vi "接口测试_20190220.vi"() -> ()   [LabVIEW 2017]
uses:
  D:/QuiKLab3.0/QuiKLabAPI.dll
panel:
  in  "启动任务":bool
  out "双击":string
  out "信号":string
  out "获取订阅的信号参数值":dbl
  in  "卸载工程 2":bool
  in  "用例运行状态":i32(listbox)
  in  "任务下用例状态":i32(listbox)
  in  "用例分类下用例":i32(listbox)
  in  "用例分类":i32(listbox)
  in  "任务分类下任务":i32(listbox)
  in  "测试任务":i32(listbox) caption="测试任务分类"
  in  "测试用例":i32(listbox)
  out "文件数量":i32
  in  "运行时参数列表":i32(listbox)
  in  "板卡设备IP":string
  out "板卡信息列表":i32(listbox)
  in  "设置的内容":string
  out "设置文件内容结果":i32
  in  "设置文件内容":bool
  out "显示的内容":string
  in  "目录":i32(listbox)=-1
  out "获取选中参数值":dbl
  in  "输入设备IP":string
  in  "下位机信息":bool
  out "下位机列表":i32(listbox)
  out "IP是否在线":i32
  out "更新信息是否成功":i32
  out "板卡类型个数":i32
  in  "字符串 3":string="00000000000000000000000000000000000000000000000000000000000000000000000000000000000000"
  out "下位机个数":i32
  in  "获得初始值列表":i32(listbox)
  in  "获得初始值":bool
  in  "输出信号列表":string(tree)
  in  "输出信号参数列表":bool
  out "项目个数":i32
  in  "工程选择：":i32(listbox)
  in  "字符串":string="00000000000000000000000000000000000000000000000000000000000000000000000000000000000000"
  in  "输入信号参数列表":bool
  in  "输入信号列表":string(tree)
  out "取消订阅":i32
  out "使用下位机返回值":i32
  in  "停止测试用例":bool
  out "StartTest":i32
  out "useTestCase":i32
  in  "执行用例":bool
  out "刷新返回结果":i32
  out "设置初始值结果":i32
  in  "设置初始值":bool
  out "发送信号结果":i32
  in  "发送信号":bool
  out "输出信号参数值":dbl
  in  "输出信号参数值":dbl
  in  "设置输出信号参数值":bool
  out "设置输出参数值":i32
  out "重置参数值":i32
  out "获取输入订阅信号参数值":dbl
  in  "重置按钮":bool
  in  "获取用例集列表":bool
  out "用例集":string(tree)
  in  "获取任务集列表":bool
  in  "任务集":string(tree)
  out "当前工程名称":string
  out "卸载工程结果":i32
  in  "卸载工程":bool
  in  "更新路径":bool
  in  "加载工程":bool
  out "导出用例相关信息结果":i32
  in  "导出工程用例相关信息":bool
  out "设置实时参数值返回值":i32
  in  "设置实时参数值":dbl
  in  "设置参数值":bool
  out "暂停和继续结果":i32
  in  "暂停按钮":bool
  out "停止任务集结果 2":i32
  out "波形图表":dbl(graph)
  in  "退出程序":bool
  in  "媒体停止按钮":bool
  in  "播放按钮":bool
  out "释放平台结果":i32
  out "卸载工程结果 2":i32
  out "停止测试用例":i32
  out "开始任务集":i32
  out "加载工程结果":i32
  out "初始化平台结果":i32
  out "错误输出":errorcluster
  out "更新路径结果":i32
  # "下位机信息"
  # "文件操作"
  # "平台初始化"
  # "测试任务执行"
  # "测试用例执行"
  # "实时监视"
  # "信号"
  # "初始值"
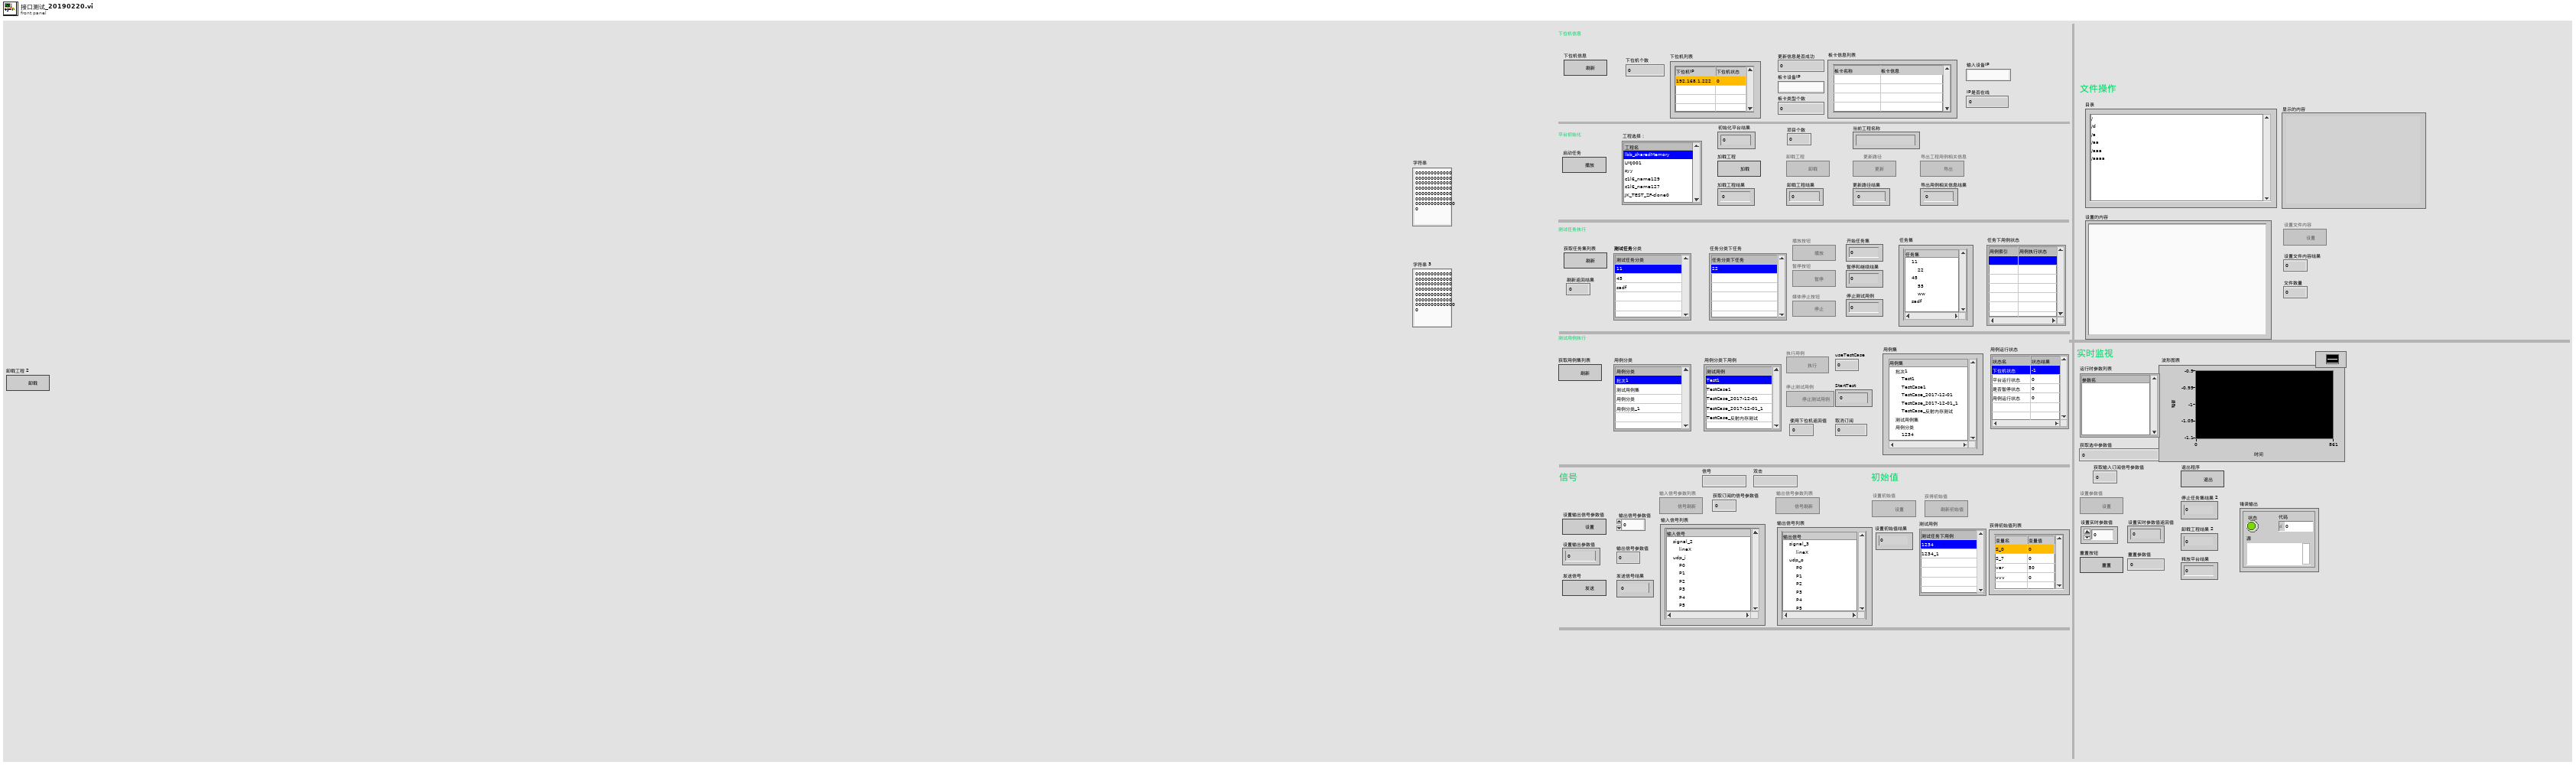
[diagram p1: front panel]
types:
  T1 = enum8{"loadPro", "unLoadPro", "updatePath", "export", "play", "pause", "stop"}
  T2 = enum8{"Enabled", "Disabled", "Disabled and Grayed Out"}
  T3 = enum8{"Enabled", "Disabled", "Disabled and Grayed Out", ""}
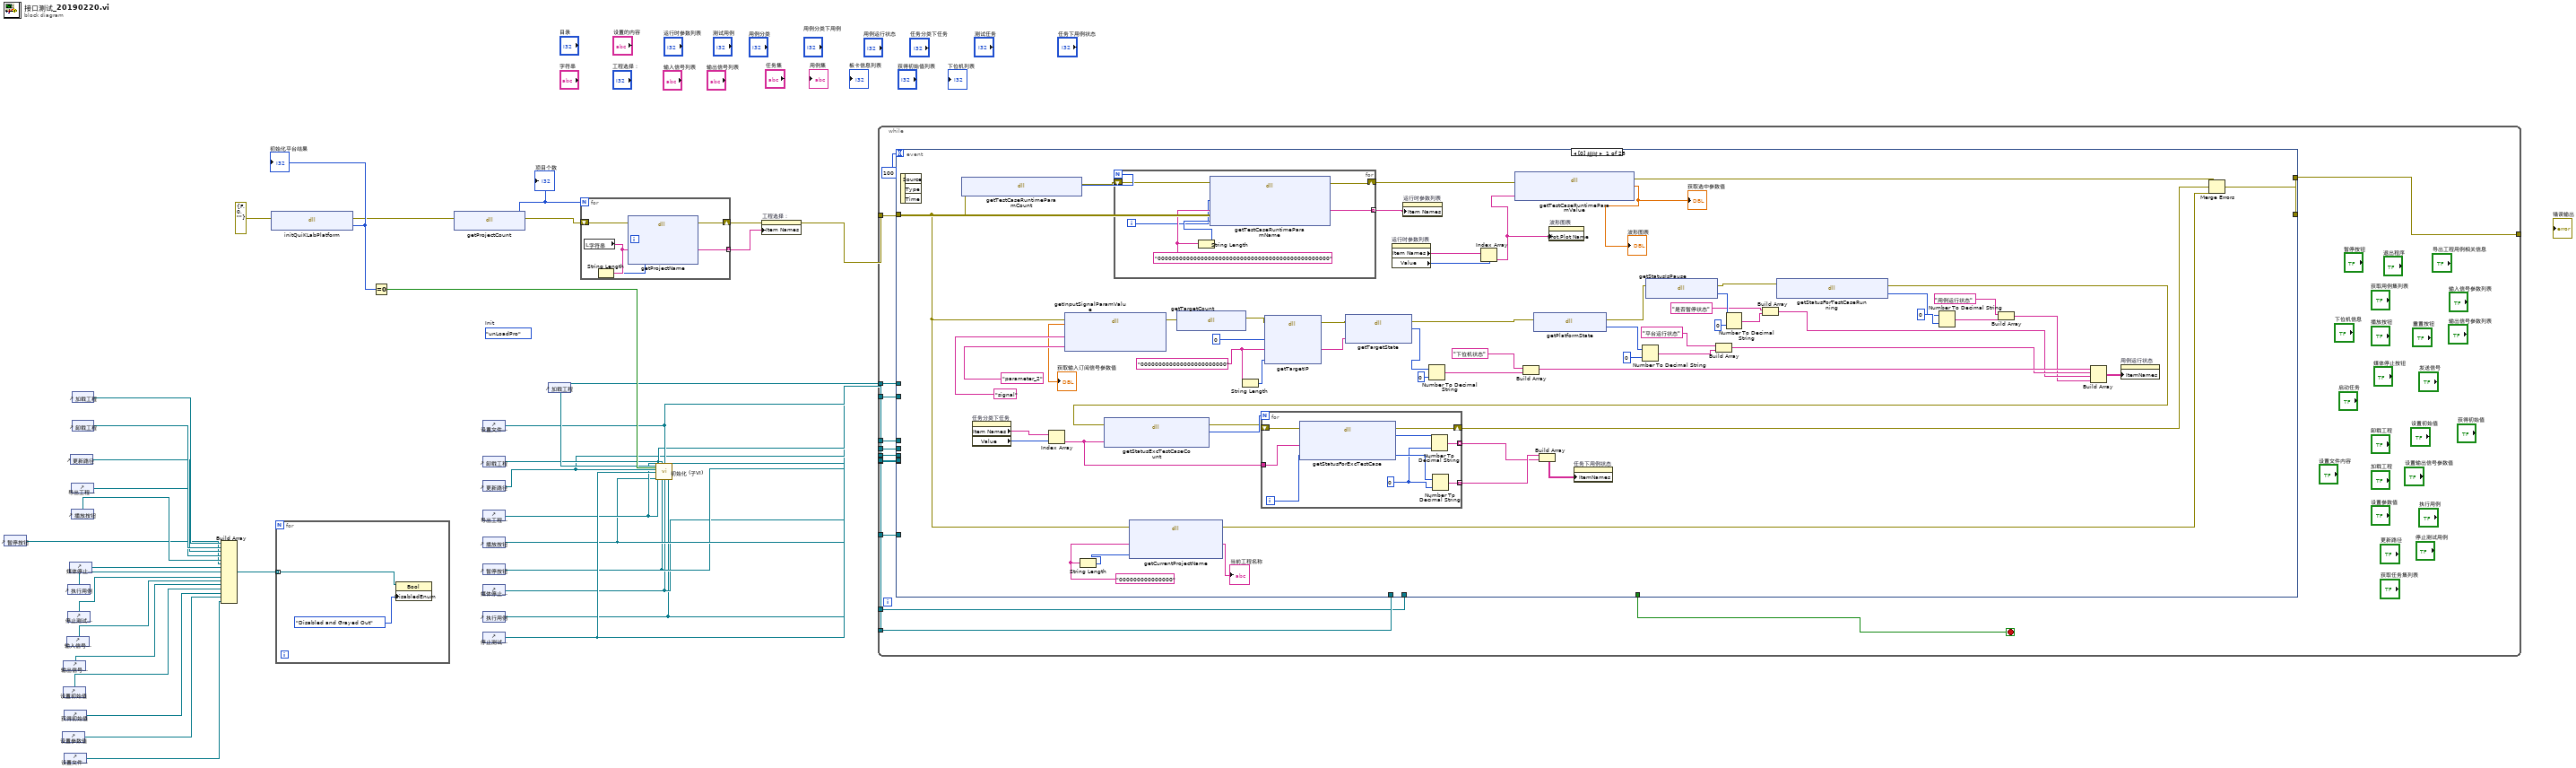
[diagram p0: block diagram]
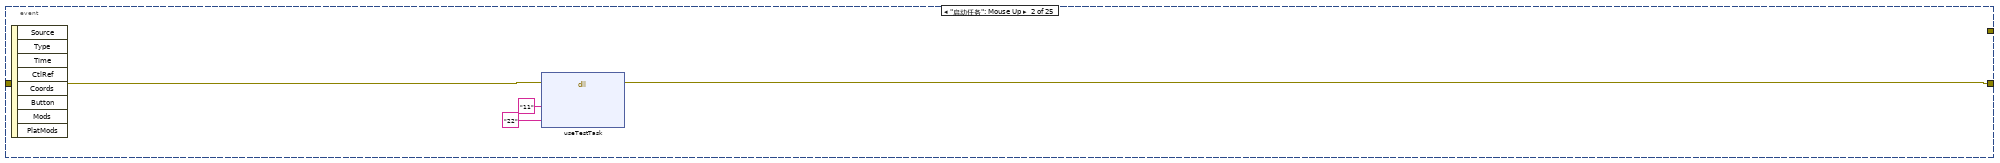
[diagram p2: hidden frame]
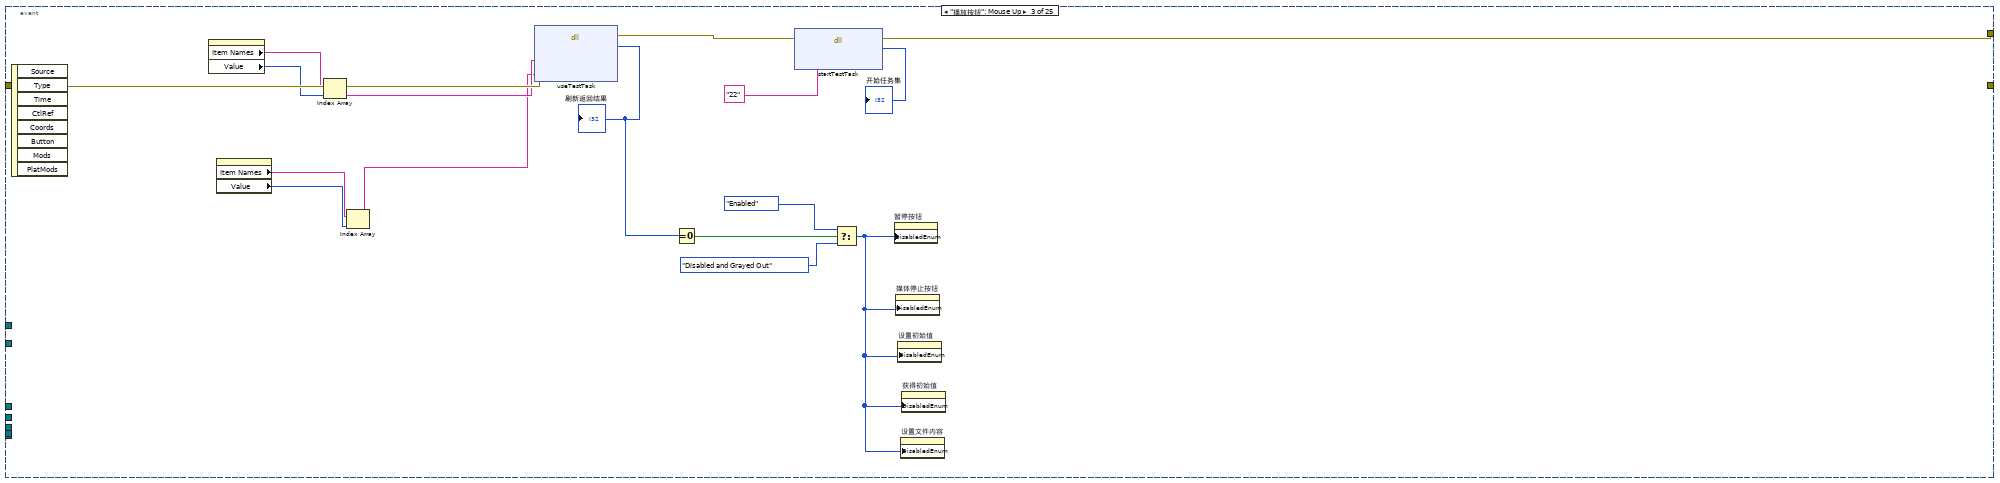
[diagram p3: hidden frame]
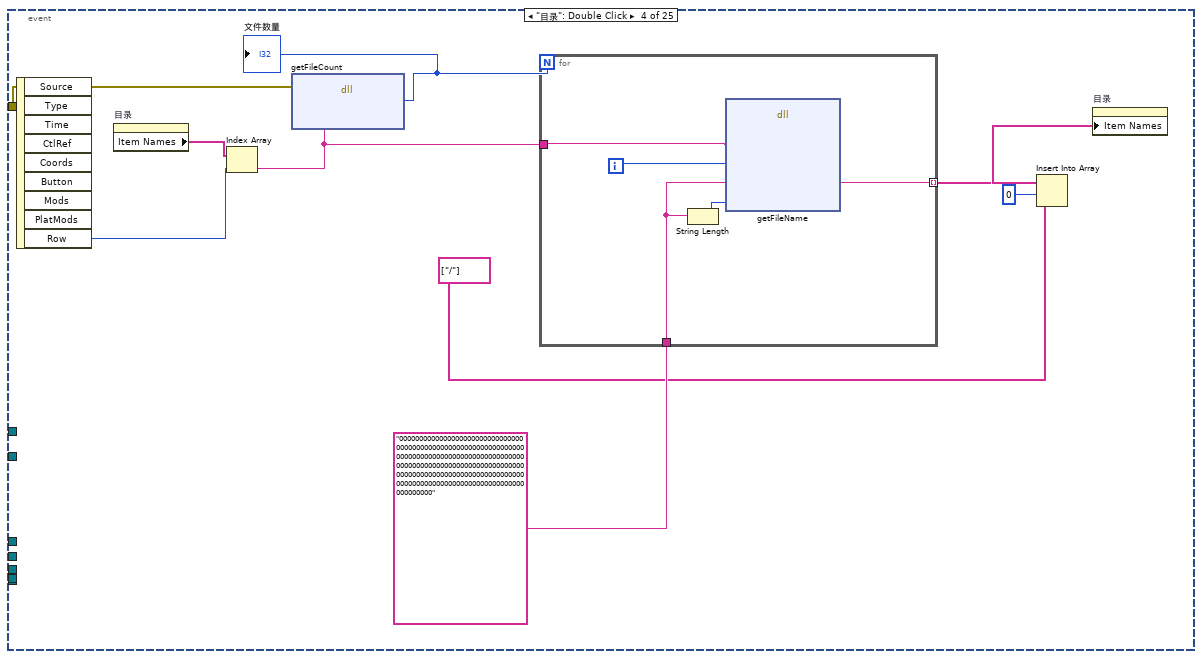
[diagram p4: hidden frame]
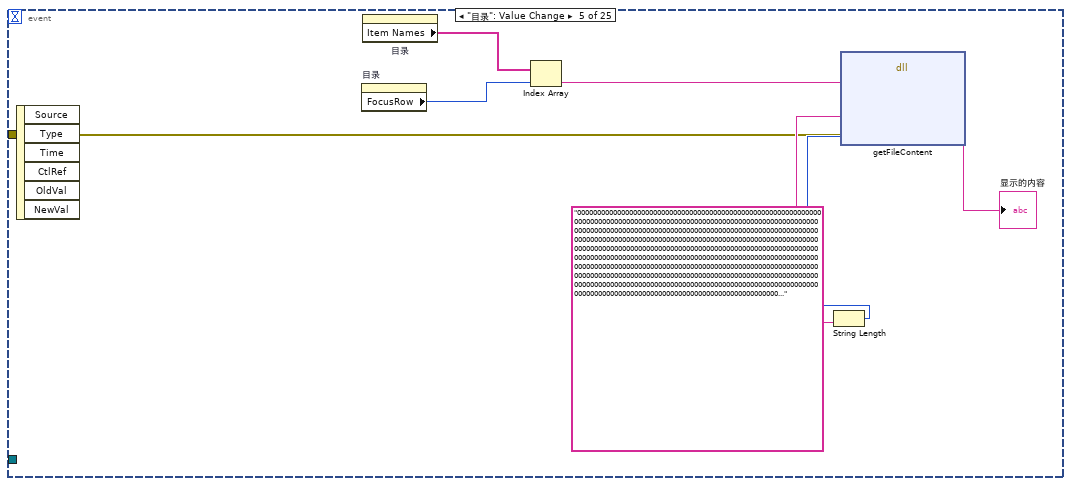
[diagram p5: hidden frame]
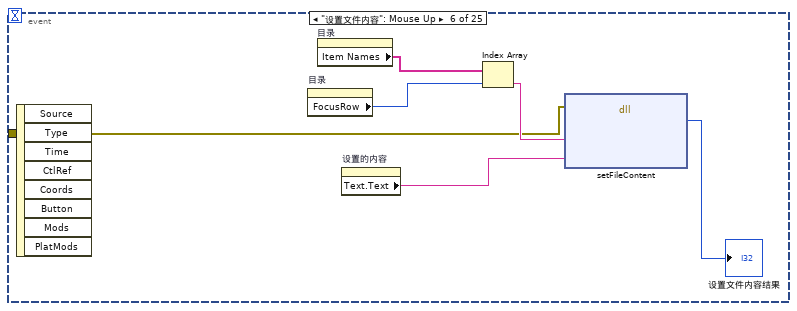
[diagram p6: hidden frame]
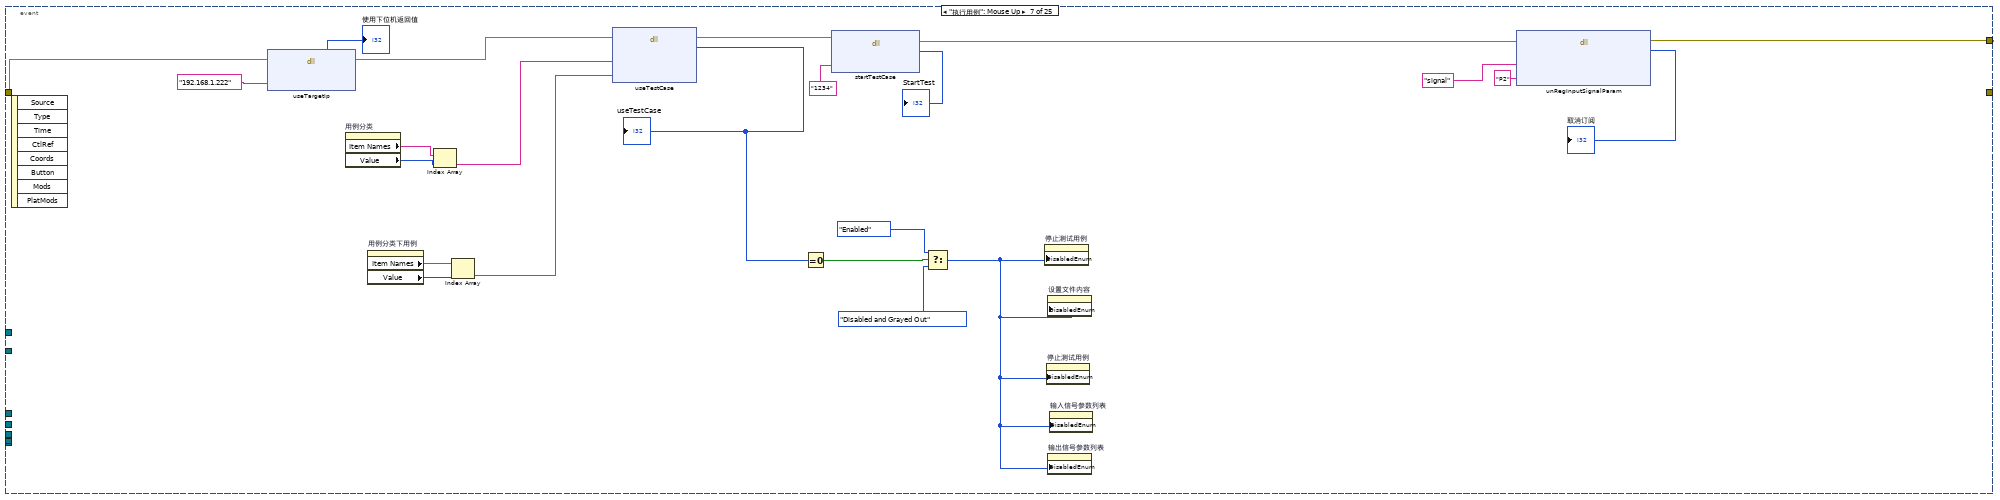
[diagram p7: hidden frame]
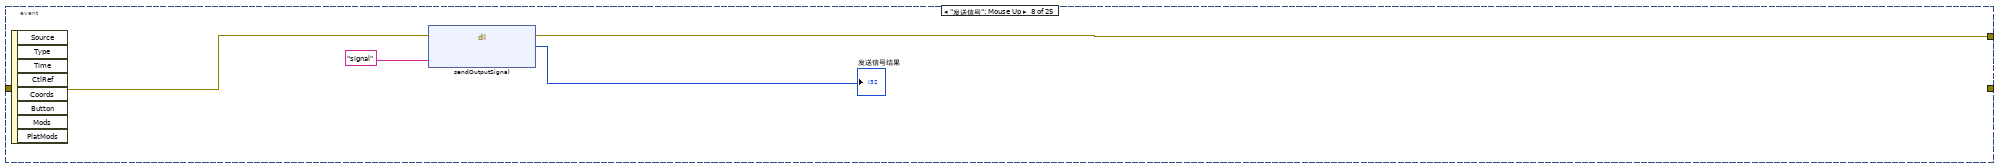
[diagram p8: hidden frame]
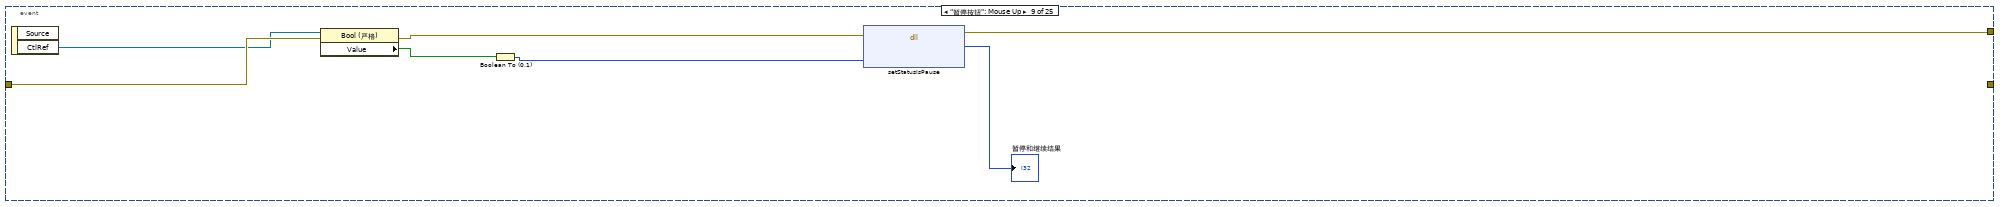
[diagram p9: hidden frame]
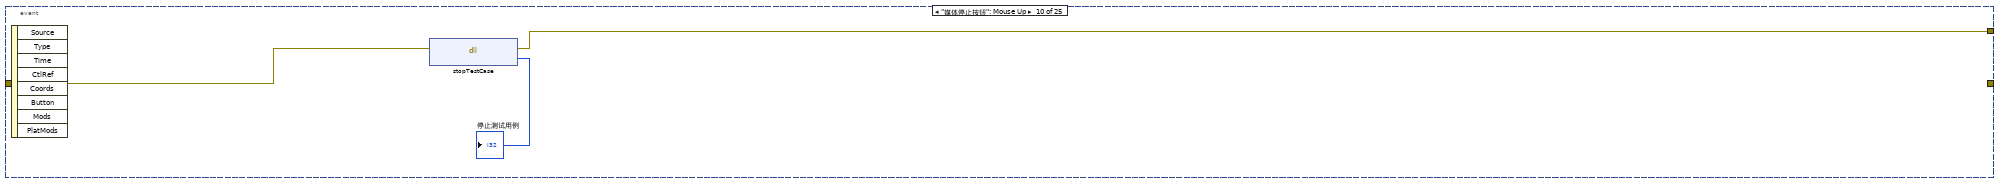
[diagram p10: hidden frame]
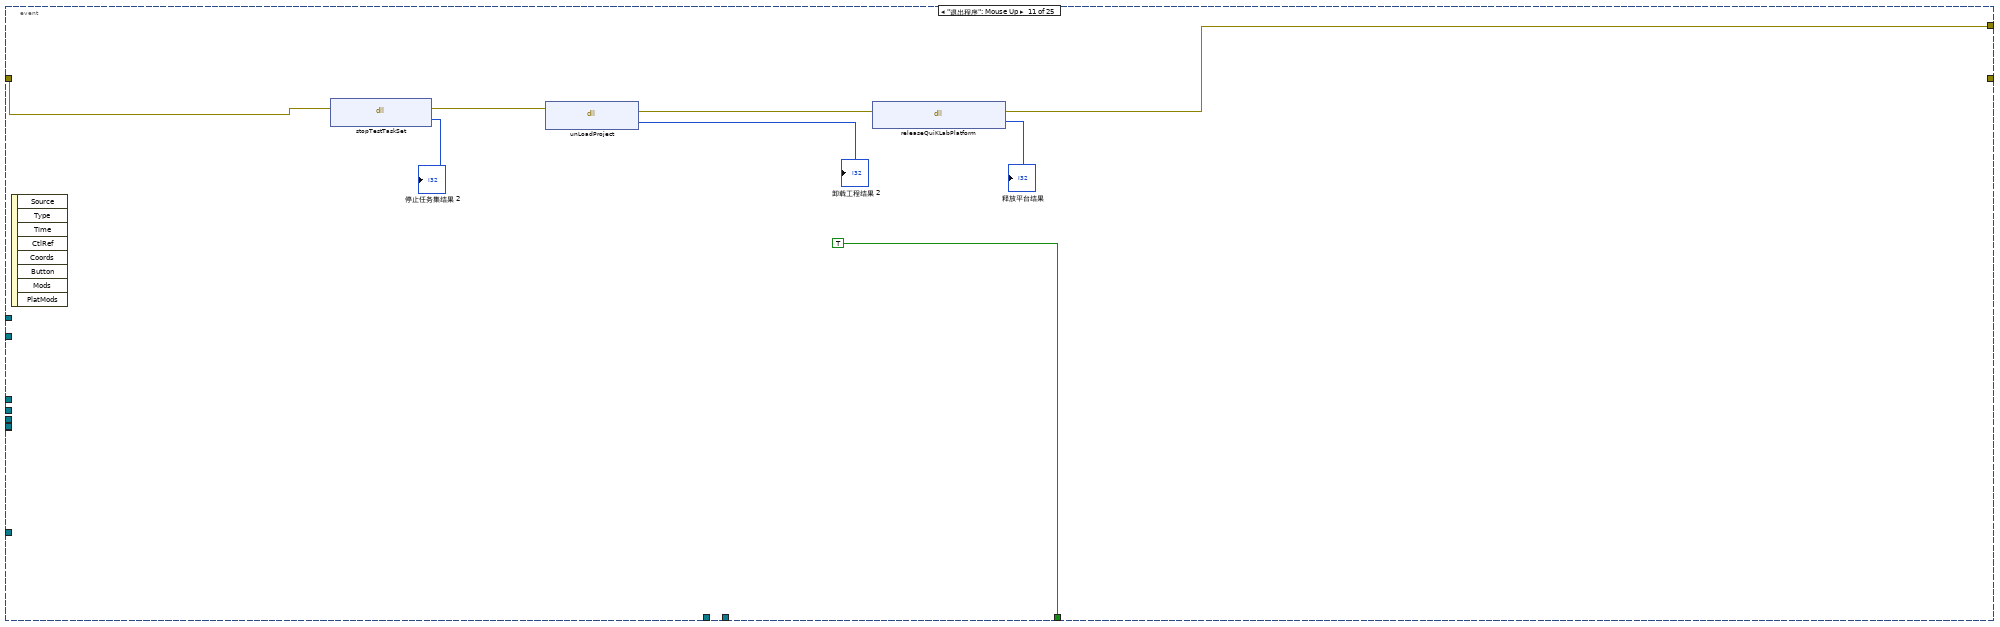
[diagram p11: hidden frame]
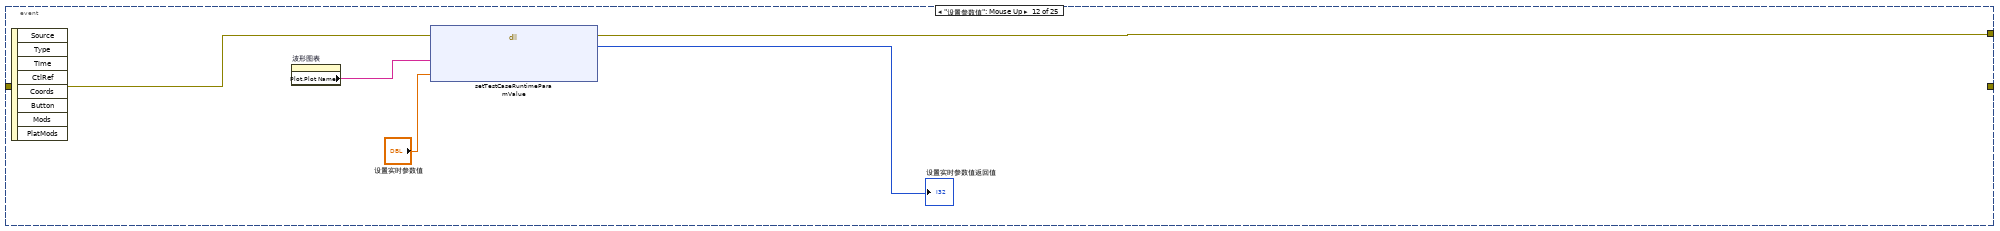
[diagram p12: hidden frame]
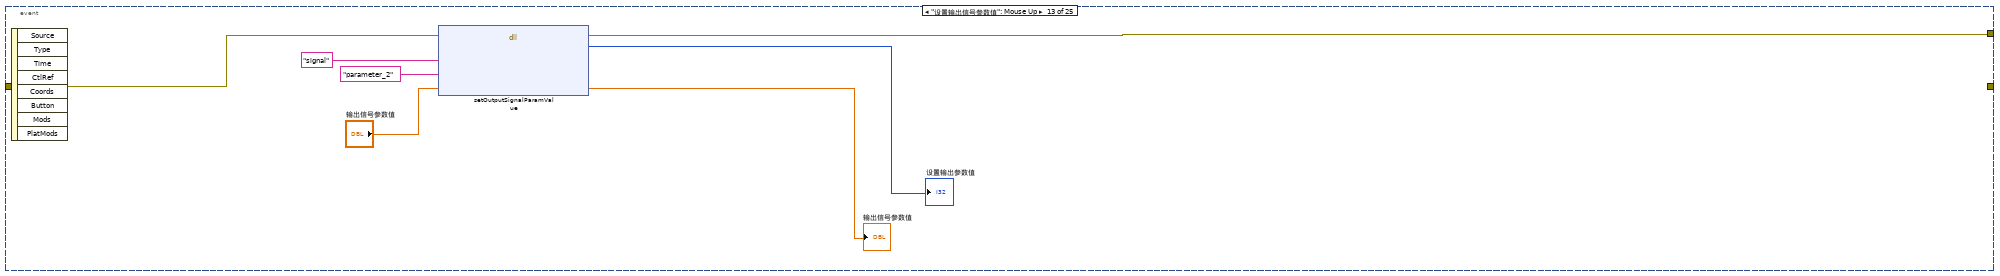
[diagram p13: hidden frame]
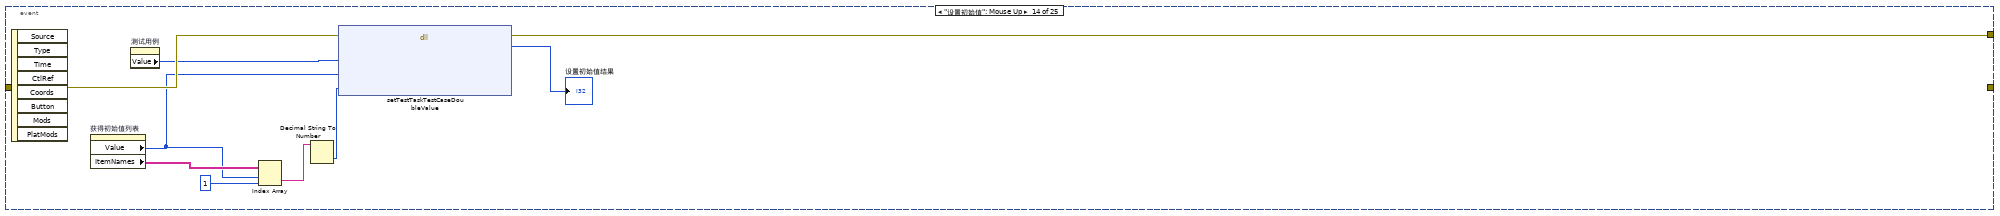
[diagram p14: hidden frame]
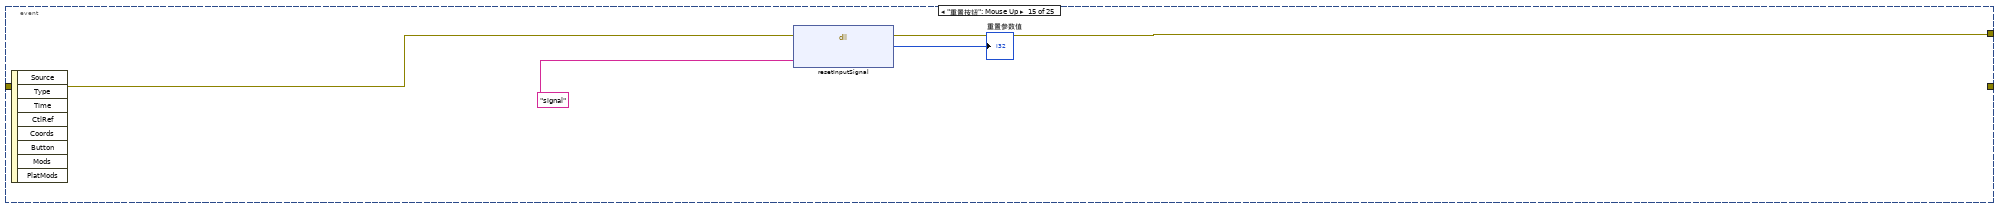
[diagram p15: hidden frame]
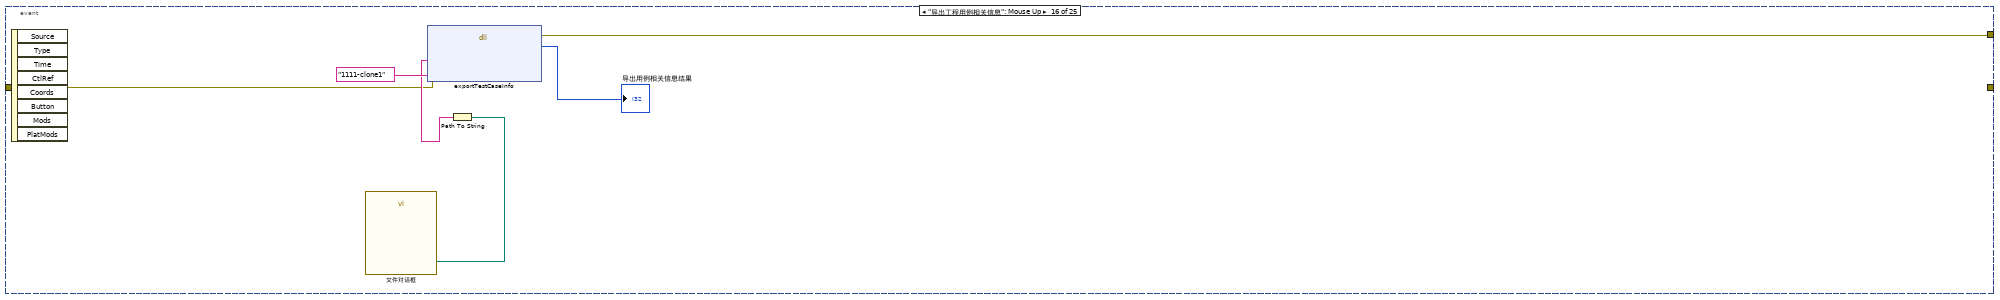
[diagram p16: hidden frame]
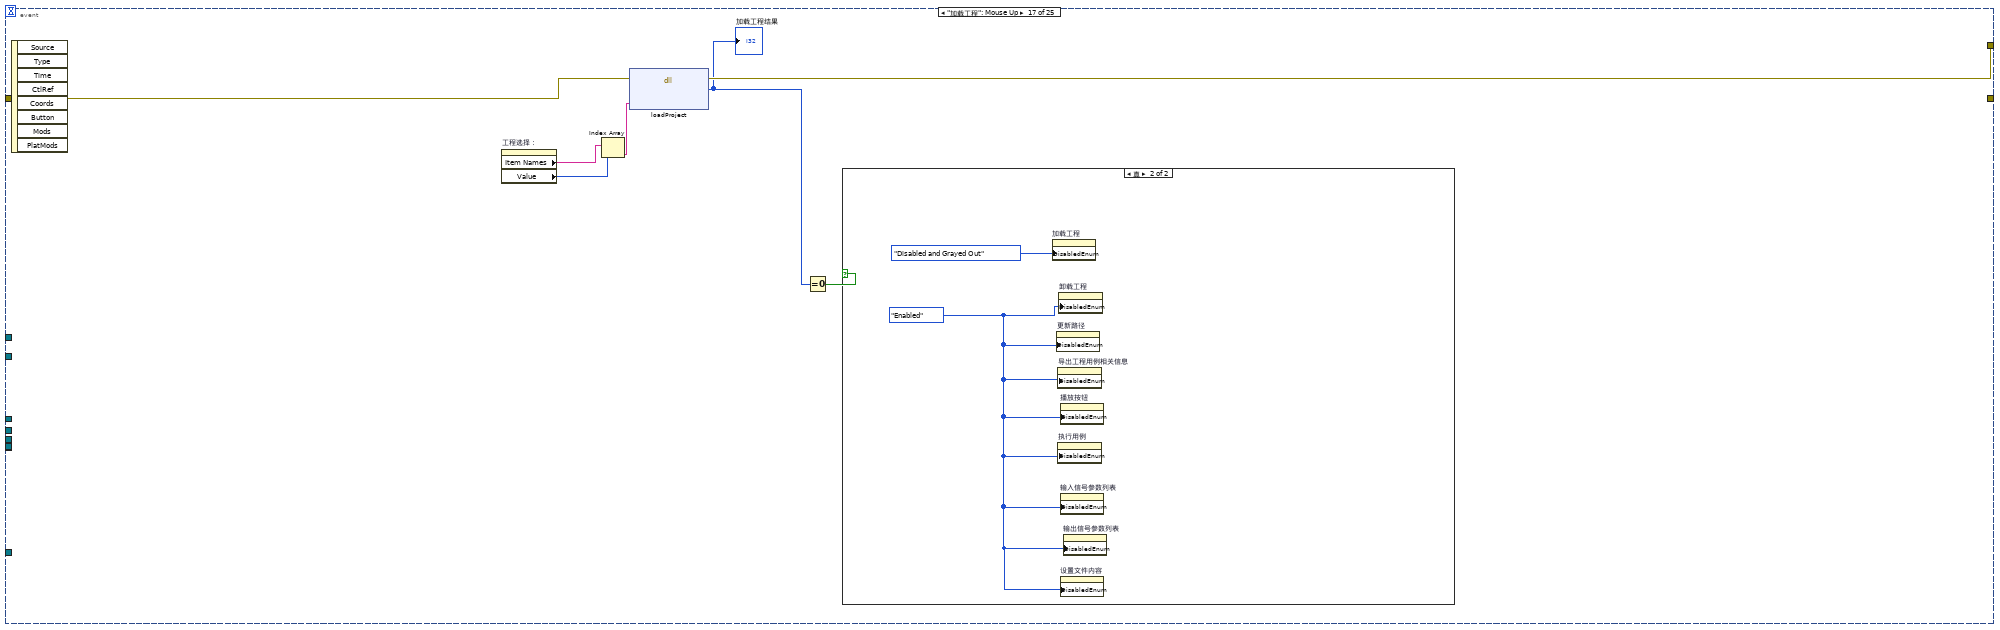
[diagram p17: hidden frame]
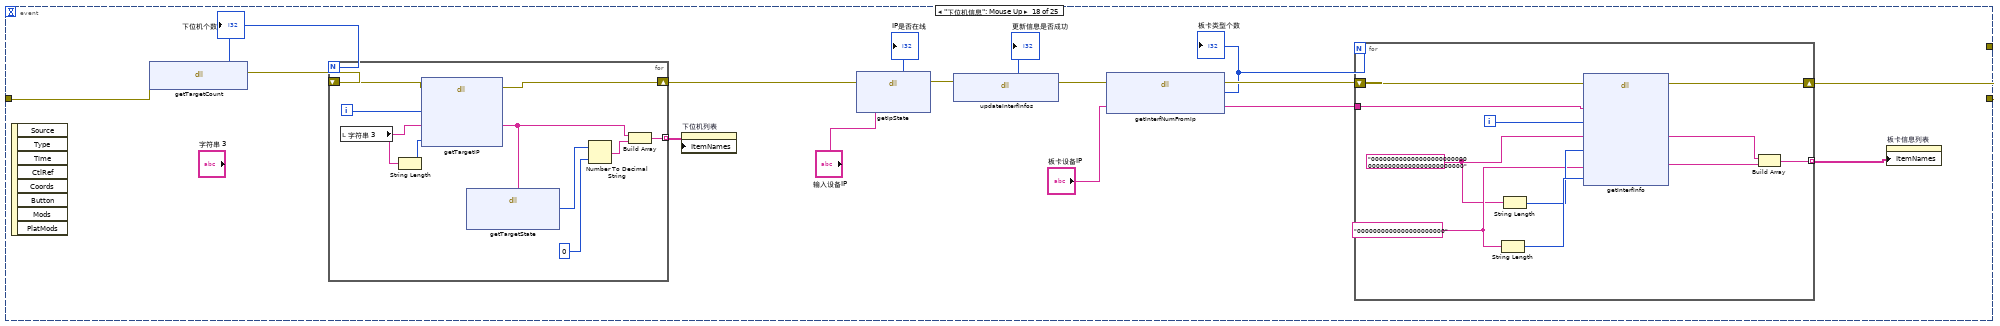
[diagram p19: hidden frame]
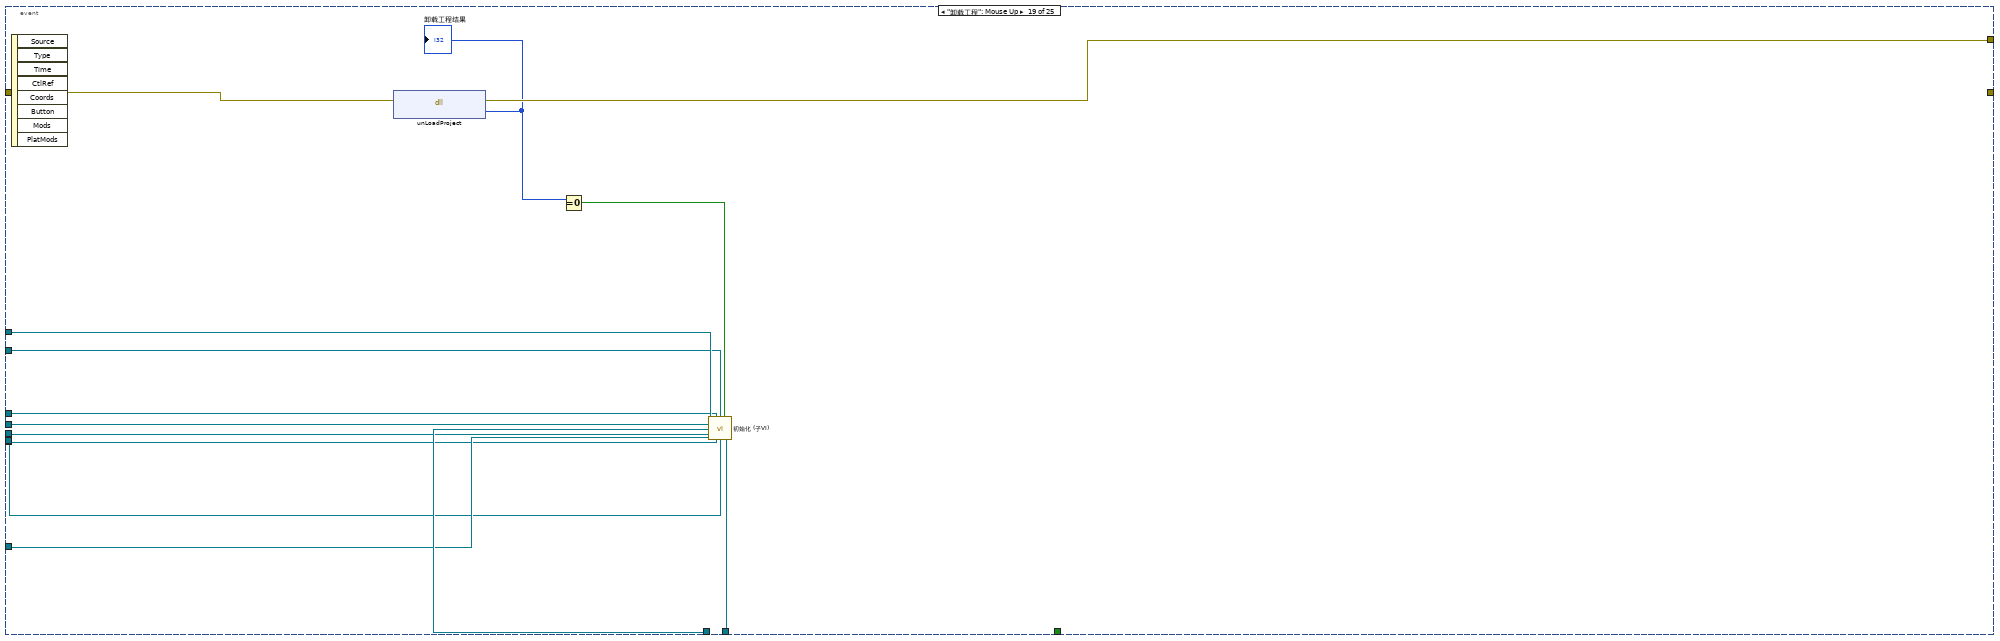
[diagram p20: hidden frame]
diagram:
  (unwired) T1."unLoadPro"  # Init
  n1 = control-ref of="暂停按钮"() -> (w1:refnum<vi>)
  n2 = control-ref of="设置参数值"() -> (w4:refnum<vi>)
  n3 = control-ref of="设置初始值"() -> (w6:refnum<vi>)
  n4 = control-ref of="输出信号参数列表"() -> (w7:refnum<vi>)
  n5 = control-ref of="获得初始值"() -> (w5:refnum<vi>)
  n6 = control-ref of="设置文件内容"() -> (w3:refnum<vi>)
  n7 = control-ref of="输入信号参数列表"() -> (w8:refnum<vi>)
  n8 = control-ref of="执行用例"() -> (w10:refnum<vi>)
  n9 = control-ref of="停止测试用例"() -> (w9:refnum<vi>)
  n10 = control-ref of="媒体停止按钮"() -> (w11:refnum<vi>)
  n11 = control-ref of="更新路径"() -> (w14:refnum<vi>)
  n12 = control-ref of="导出工程用例相关信息"() -> (w13:refnum<vi>)
  n13 = control-ref of="播放按钮"() -> (w12:refnum<vi>)
  n14 = control-ref of="加载工程"() -> (w16:refnum<vi>)
  n15 = control-ref of="卸载工程"() -> (w15:refnum<vi>)
  n16 = Build Array(w16, w15, w14, w13, w12, w1, w11, w10, w9, w8, w7, w6, w5, w4, w3) -> (w2:refnum<vi>[])
  n17 = dll-call lib="D:/QuiKLab3.0/QuiKLabAPI.dll" fn="initQuiKLabPlatform"(error in=errorcluster {"status"=FALSE, "code"=0, "source"=""} ("错误输入（无错误）")) -> (error out=w17:errorcluster, "初始化平台结果"=w29:i32)  [unwired: 2 in, 1 out]
  "初始化平台结果" <- w29
  n18 = for {
    tunnel: w2 -> [w36] mode=indexing
    n19 = property on="属性节点" class="Bool"(reference=w36, "DisabledEnum"=T2."Disabled and Grayed Out" ("Disable")) -> ()  [unwired: 1 in, 2 out]
  }
  n20 = Equal To 0?(x=w29) -> (x = 0?=w28:bool)
  n21 = dll-call lib="D:/QuiKLab3.0/QuiKLabAPI.dll" fn="getProjectCount"(error in=w17) -> (error out=w32:errorcluster, "项目个数"=w34:i32)  [unwired: 2 in, 1 out]
  "项目个数" <- w34
  n22 = control-ref of="设置文件内容"() -> (w26:refnum<vi>)
  n23 = control-ref of="卸载工程"() -> (w25:refnum<vi>)
  n24 = control-ref of="更新路径"() -> (w24:refnum<vi>)
  n25 = control-ref of="导出工程用例相关信息"() -> (w22:refnum<vi>)
  n26 = control-ref of="播放按钮"() -> (w21:refnum<vi>)
  n27 = control-ref of="暂停按钮"() -> (w20:refnum<vi>)
  n28 = control-ref of="媒体停止按钮"() -> (w19:refnum<vi>)
  n29 = control-ref of="执行用例"() -> (w18:refnum<vi>)
  n30 = control-ref of="停止测试用例"() -> (w23:refnum<vi>)
  n31 = control-ref of="加载工程"() -> (w27:refnum<vi>)
  n32 = for {
    N: w34 -> [_]
    shift-right: [w43] -> w33
    shift-left: w32 -> [w38]
    tunnel: [w41] -> w35 mode=indexing
    i -> [w42]
    n33 = local read "字符串"() -> (w40:string)
    n34 = String Length(string=w40) -> (length=w39:i32)
    n35 = dll-call lib="D:/QuiKLab3.0/QuiKLabAPI.dll" fn="getProjectName"(error in=w38, "项目索引"=w42, "项目名"=w40, "长度"=w39) -> (error out=w43:errorcluster, "项目名"=w41:string)  [unwired: 5 in, 1 out]
  }
  n36 = call "初始化 (子VI).vi"("Boolean输入"=w27, "卸载工程"=w25, "设置文件内容"=w26, "布尔"=w28, "更新路径"=w24, "停止测试用例"=w23, "导出工程用例相关信息"=w22, "播放按钮"=w21, "暂停按钮"=w20, "媒体停止按钮"=w19, "执行用例"=w18) -> ()  [unwired: 5 in]
  n37 = property on="工程选择：" class="LstBox (严格)"(error in=w33, "Item Names"=w35) -> (error out=w31:errorcluster)  [unwired: 1 in, 1 out]
  n38 = while {
    tunnel: [w55] -> _
    tunnel: w31 -> [w56]
    tunnel: w27 -> [w53]
    tunnel: w26 -> [w52]
    tunnel: w25 -> [w51]
    tunnel: w24 -> [w50]
    tunnel: w23 -> [w49]
    tunnel: w22 -> [w48]
    tunnel: w21 -> [w47]
    tunnel: w20 -> [w46]
    tunnel: w19 -> [w45]
    tunnel: w18 -> [w44]
    stop <- w57 stop-if-true
    n39 = event shown="[0] 超时" {
      selector: _ -> [_ _ _ _ _ _ _ _ _ _ _ _ _ _ _ _ _ _ _ _ _ _ _ _ _]
      dyn-events: _ -> [_ _ _ _ _ _ _ _ _ _ _ _ _ _ _ _ _ _ _ _ _ _ _ _ _]
      timeout: 100 -> [_ _ _ _ _ _ _ _ _ _ _ _ _ _ _ _ _ _ _ _ _ _ _ _ _]
      tunnel: [w114 _ w136 _ _ _ w195 w204 w213 w215 w221 w226 w234 w243 w248 w251 w258 _ w314 w316 w327 w355 w384 w415 _] -> _
      tunnel: [_ _ _ _ _ _ _ _ _ _ TRUE _ _ _ _ _ _ _ _ _ _ _ _ _ _] -> w57
      tunnel: w56 -> [w105 w135 w149 w161 w167 w174 w198 w205 w211 w214 w218 w229 w236 w245 w249 w250 w262 w275 w315 w317 w330 w358 w387 w419 w450]
      tunnel: [_ w134 _ _ _ _ _ _ _ _ _ _ _ _ _ _ _ w270 _ _ _ _ _ _ w444] -> w55
      tunnel: w53 -> [_ _ _ _ _ _ _ _ _ _ _ _ _ _ _ _ _ _ w311 _ _ _ _ _ _]
      tunnel: w52 -> [_ _ _ _ _ _ _ _ _ _ _ _ _ _ _ _ _ _ w310 _ _ _ _ _ _]
      tunnel: w51 -> [_ _ _ _ _ _ _ _ _ _ _ _ _ _ _ _ _ _ w309 _ _ _ _ _ _]
      tunnel: w50 -> [_ _ _ _ _ _ _ _ _ _ _ _ _ _ _ _ _ _ w308 _ _ _ _ _ _]
      tunnel: w49 -> [_ _ _ _ _ _ _ _ _ _ _ _ _ _ _ _ _ _ w307 _ _ _ _ _ _]
      tunnel: w48 -> [_ _ _ _ _ _ _ _ _ _ _ _ _ _ _ _ _ _ w306 _ _ _ _ _ _]
      tunnel: w47 -> [_ _ _ _ _ _ _ _ _ _ _ _ _ _ _ _ _ _ w305 _ _ _ _ _ _]
      tunnel: w46 -> [_ _ _ _ _ _ _ _ _ _ _ _ _ _ _ _ _ _ w304 _ _ _ _ _ _]
      tunnel: w45 -> [_ _ _ _ _ _ _ _ _ _ _ _ _ _ _ _ _ _ w303 _ _ _ _ _ _]
      tunnel: w44 -> [_ _ _ _ _ _ _ _ _ _ _ _ _ _ _ _ _ _ w302 _ _ _ _ _ _]
      event Timeout {
        w59 = "000000000000000000000000" ("IP值")
        w110 = "000000000000000" ("当前工程名称")
        n40 = event-data() -> ()  [unwired: 1 in, 3 out]
        n41 = dll-call lib="D:/QuiKLab3.0/QuiKLabAPI.dll" fn="getTestCaseRuntimeParamCount"(error in=w105) -> (error out=w103:errorcluster, "获取运行时参数数量"=w104:i32)  [unwired: 2 in, 1 out]
        n42 = property on="任务分类下任务" class="LstBox (严格)"() -> ("Item Names"=w97:string[], "Value"=w96:i32)  [unwired: 2 in, 2 out]
        n43 = Index Array(array=w97, index=w96) -> (element=w91:string)
        n44 = dll-call lib="D:/QuiKLab3.0/QuiKLabAPI.dll" fn="getInputSignalParamValue"(error in=w105, "信号名"="signal" ("任务名"), "参数名"="parameter_2" ("任务名")) -> (error out=w64:errorcluster, "获取订阅的信号参数值"=→"获取输入订阅信号参数值":dbl)  [unwired: 4 in, 1 out]
        n45 = String Length(string=w110) -> (length=w111:i32)
        n46 = for {
          N: w104 -> [_]
          shift-right: [w126] -> w99
          shift-left: w103 -> [w128]
          tunnel: [w127] -> w98 mode=indexing
          i -> [w129]
          w131 = "000000000000000000000000000000000000000000000000" ("参数名称")
          n47 = String Length(string=w131) -> (length=w130:i32)
          n48 = dll-call lib="D:/QuiKLab3.0/QuiKLabAPI.dll" fn="getTestCaseRuntimeParamName"(error in=w128, "参数索引"=w129, "参数名称"=w131, "参数名称长度"=w130) -> (error out=w126:errorcluster, "参数名称"=w127:string)  [unwired: 5 in, 1 out]
        }
        n49 = dll-call lib="D:/QuiKLab3.0/QuiKLabAPI.dll" fn="getCurrentProjectName"(error in=w105, "当前工程名称"=w110, "长度"=w111) -> (error out=w109:errorcluster, "当前工程名称"=→"当前工程名称":string)  [unwired: 4 in, 1 out]
        n50 = dll-call lib="D:/QuiKLab3.0/QuiKLabAPI.dll" fn="getTargetCount"(error in=w64) -> (error out=w61:errorcluster)  [unwired: 3 in, 1 out]
        n51 = String Length(string=w59) -> (length=w58:i32)
        n52 = dll-call lib="D:/QuiKLab3.0/QuiKLabAPI.dll" fn="getTargetIP"(error in=w61, "索引"=0, "IP值"=w59, "IP长度"=w58) -> (error out=w60:errorcluster, "IP值"=w62:string)  [unwired: 5 in, 1 out]
        n53 = dll-call lib="D:/QuiKLab3.0/QuiKLabAPI.dll" fn="getTargetState"(error in=w60, "下位机IP"=w62) -> (error out=w77:errorcluster, "下位机状态"=w65:i32)  [unwired: 3 in, 1 out]
        n54 = property on="运行时参数列表" class="LstBox (严格)"() -> ("Item Names"=w102:string[], "Value"=w101:i32)  [unwired: 2 in, 2 out]
        n55 = property on="运行时参数列表" class="LstBox (严格)"("Item Names"=w98) -> ()  [unwired: 2 in, 2 out]
        n56 = Number To Decimal String(number=w65, width (-)=i16 0 ("宽度(-)")) -> (decimal integer string=w70:string)
        n57 = Index Array(array=w102, index=w101) -> (element=w100:string)
        n58 = dll-call lib="D:/QuiKLab3.0/QuiKLabAPI.dll" fn="getTestCaseRuntimeParamValue"(error in=w99, "参数名"=w100) -> (error out=w113:errorcluster, "获取参数值"=→"波形图表" →"获取选中参数值":dbl)  [unwired: 3 in, 1 out]
        n59 = Build Array("下位机状态" ("任务名"), w70) -> (w69:string[])
        n60 = dll-call lib="D:/QuiKLab3.0/QuiKLabAPI.dll" fn="getPlatformState"(error in=w77) -> (error out=w78:errorcluster, "获取平台运行状态"=w76:i32)  [unwired: 2 in, 1 out]
        n61 = property on="波形图表" class="WFChart (严格)"("Plot.Plot Name"=w100) -> ()  [unwired: 2 in, 2 out]
        n62 = Number To Decimal String(number=w76, width (-)=i16 0 ("宽度(-)")) -> (decimal integer string=w73:string)
        n63 = dll-call lib="D:/QuiKLab3.0/QuiKLabAPI.dll" fn="getStatusIsPause"(error in=w78) -> (error out=w115:errorcluster, "是否暂停状态"=w87:i32)  [unwired: 2 in, 1 out]
        n64 = Build Array("平台运行状态" ("任务名"), w73) -> (w68:string[])
        n65 = Number To Decimal String(number=w87, width (-)=i16 0 ("宽度(-)")) -> (decimal integer string=w85:string)
        n66 = Build Array("是否暂停状态" ("任务名"), w85) -> (w67:string[])
        n67 = dll-call lib="D:/QuiKLab3.0/QuiKLabAPI.dll" fn="getStatusForTestCaseRunning"(error in=w115) -> (error out=w95:errorcluster, "用例运行状态"=w82:i32)  [unwired: 2 in, 1 out]
        n68 = dll-call lib="D:/QuiKLab3.0/QuiKLabAPI.dll" fn="getStatusExcTestCaseCount"(error in=w95, "任务名"=w91) -> (error out=w93:errorcluster, "获取执行中的测试用例个数"=w94:i32)  [unwired: 3 in, 1 out]
        n69 = for {
          N: w94 -> [_]
          shift-right: [w124] -> w92
          shift-left: w93 -> [w125]
          tunnel: w91 -> [w122]
          tunnel: [w118] -> w89 mode=indexing
          tunnel: [w117] -> w88 mode=indexing
          i -> [w123]
          w119 = i16 0 ("宽度(-)")
          n70 = dll-call lib="D:/QuiKLab3.0/QuiKLabAPI.dll" fn="getStatusForExcTestCase"(error in=w125, "任务名"=w122, "任务用例索引"=w123) -> (error out=w124:errorcluster, "某个用例状态"=w120:i32, "任务用例索引"=w121:i32)  [unwired: 3 in, 1 out]
          n71 = Number To Decimal String(number=w120, width (-)=w119) -> (decimal integer string=w117:string)
          n72 = Number To Decimal String(number=w121, width (-)=w119) -> (decimal integer string=w118:string)
        }
        n73 = Build Array(w89, w88) -> (w90:string[][])
        n74 = property on="任务下用例状态" class="MCListbox (严格)"("ItemNames"=w90) -> ()  [unwired: 2 in, 2 out]
        n75 = Number To Decimal String(number=w82, width (-)=i16 0 ("宽度(-)")) -> (decimal integer string=w80:string)
        n76 = Build Array("用例运行状态" ("任务名"), w80) -> (w66:string[])
        n77 = Build Array(w69, w68, w67, w66) -> (w79:string[][])
        n78 = property on="用例运行状态" class="MCListbox (严格)"("ItemNames"=w79) -> ()  [unwired: 2 in, 2 out]
        n79 = Merge Errors(w113, w92, w109) -> (w114:errorcluster)
      }
      event "启动任务": Mouse Up {
        n80 = event-data() -> ()  [unwired: 1 in, 8 out]
        n81 = dll-call lib="D:/QuiKLab3.0/QuiKLabAPI.dll" fn="useTestTask"(error in=w135, "任务集名"="11", "任务名"="22") -> (error out=w134:errorcluster)  [unwired: 5 in, 1 out]
      }
      event "播放按钮": Mouse Up {
        n82 = event-data() -> ()  [unwired: 1 in, 8 out]
        n83 = property on="测试任务" class="LstBox (严格)"() -> ("Item Names"=w147:string[], "Value"=w146:i32)  [unwired: 2 in, 2 out]
        n84 = property on="任务分类下任务" class="LstBox (严格)"() -> ("Item Names"=w144:string[], "Value"=w143:i32)  [unwired: 2 in, 2 out]
        n85 = Index Array(array=w147, index=w146) -> (element=w145:string)
        n86 = Index Array(array=w144, index=w143) -> (element=w142:string)
        n87 = dll-call lib="D:/QuiKLab3.0/QuiKLabAPI.dll" fn="useTestTask"(error in=w149, "任务集名"=w145, "任务名"=w142) -> (error out=w148:errorcluster, "useTestTask"=w141:i32)  [unwired: 4 in, 1 out]
        "刷新返回结果" <- w141
        n88 = Equal To 0?(x=w141) -> (x = 0?=w140:bool)
        n89 = dll-call lib="D:/QuiKLab3.0/QuiKLabAPI.dll" fn="startTestTask"(error in=w148, "任务集名"="22") -> (error out=w136:errorcluster, "开始任务集"=→"开始任务集":i32)  [unwired: 3 in, 1 out]
        n90 = Select(t=T3."Enabled" ("Disable"), s=w140, f=T3."Disabled and Grayed Out" ("Disable")) -> (s? t:f=w137:T3)
        n91 = property on="暂停按钮" class="Bool (严格)"("DisabledEnum"=w137) -> ()  [unwired: 2 in, 2 out]
        n92 = property on="媒体停止按钮" class="Bool"("DisabledEnum"=w137) -> ()  [unwired: 2 in, 2 out]
        n93 = property on="设置初始值" class="Bool"("DisabledEnum"=w137) -> ()  [unwired: 2 in, 2 out]
        n94 = property on="设置文件内容" class="Bool"("DisabledEnum"=w137) -> ()  [unwired: 2 in, 2 out]
        n95 = property on="获得初始值" class="Bool"("DisabledEnum"=w137) -> ()  [unwired: 2 in, 2 out]
      }
      event "目录": Double Click {
        n96 = event-data() -> ("Row"=w154:i32)  [unwired: 1 in, 8 out]
        n97 = property on="目录" class="LstBox (严格)"() -> ("Item Names"=w155:string[])  [unwired: 2 in, 2 out]
        n98 = Index Array(array=w155, index=w154) -> (element=w153:string)
        n99 = dll-call lib="D:/QuiKLab3.0/QuiKLabAPI.dll" fn="getFileCount"(error in=w161, "目录"=w153) -> ("文件数量结果"=w160:i32)  [unwired: 3 in, 2 out]
        "文件数量" <- w160
        n100 = for {
          N: w160 -> [_]
          tunnel: "00000000000000000000000000000000000000000000000000000000000000000000000000000000000000000000000000000000000000000000000000000000000000000000000000000000000000000000000000000000000000000000000000000000" -> [w165]
          tunnel: [w163] -> w156 mode=indexing
          tunnel: w153 -> [w162]
          i -> [w166]
          n101 = String Length(string=w165) -> (length=w164:i32)
          n102 = dll-call lib="D:/QuiKLab3.0/QuiKLabAPI.dll" fn="getFileName"("目录"=w162, "文件索引"=w166, "文件名"=w165, "文件名大小"=w164) -> ("文件名"=w163:string)  [unwired: 7 in, 2 out]
        }
        n103 = Insert Into Array(array=w156, index=0 ("索引"), new element=string[] ["/"] ("项名")) -> (w157:string[])
        n104 = property on="目录" class="LstBox (严格)"("Item Names"=w157) -> ()  [unwired: 2 in, 2 out]
      }
      event "目录": Value Change {
        w172 = "000000000000000000000000000000000000000000000000000000000000000000000000000000000000000000000000000000000000000000000000000000000000000000000000000000000000000000000000000000000000000000000000000000000000000000000000000000000000000000000000000000000000000000000000000000000000000000000000000000000000000000000000000000000000000000000000000000000000000000000000000000000000000000000000000000000000000000000000000000000000000000000000000000000000000000000000000000000000000000000000000000000000000000000000000000000000000000000000000000000000000000000000000000000000000000000000000000000000000000000000000000000000000000000000000000000000000000000000000000000000000000000000000000000000000000000000000000000000000000000000000000000000000000000000000000000000000000000000000000000000000000000000000000000000000000000000000000000000000000000000000000000000000000000000000000000000000000000000000000000000000000000000000000000000000000000000000000000000000000000000000000000000000000000000000000000000000000000000000000000000000000000000000000000000000000000000000000000000000000000000000000000000000000000000000000000000000000000000000000000000000000000000"
        n105 = event-data() -> ()  [unwired: 1 in, 6 out]
        n106 = property on="目录" class="LstBox (严格)"() -> ("FocusRow"=w169:i32)  [unwired: 2 in, 2 out]
        n107 = property on="目录" class="LstBox (严格)"() -> ("Item Names"=w170:string[])  [unwired: 2 in, 2 out]
        n108 = Index Array(array=w170, index=w169) -> (element=w168:string)
        n109 = String Length(string=w172) -> (length=w173:i32)
        n110 = dll-call lib="D:/QuiKLab3.0/QuiKLabAPI.dll" fn="getFileContent"(error in=w167, "文件名"=w168, "内容"=w172, "内容大小"=w173) -> ("内容"=→"显示的内容":string)  [unwired: 5 in, 2 out]
      }
      event "设置文件内容": Mouse Up {
        n111 = event-data() -> ()  [unwired: 1 in, 8 out]
        n112 = property on="目录" class="LstBox (严格)"() -> ("FocusRow"=w177:i32)  [unwired: 2 in, 2 out]
        n113 = property on="目录" class="LstBox (严格)"() -> ("Item Names"=w178:string[])  [unwired: 2 in, 2 out]
        n114 = property on="设置的内容" class="Str"() -> ("Text.Text"=w179:string)  [unwired: 2 in, 2 out]
        n115 = Index Array(array=w178, index=w177) -> (element=w176:string)
        n116 = dll-call lib="D:/QuiKLab3.0/QuiKLabAPI.dll" fn="setFileContent"(error in=w174, "文件名"=w176, "文件内容"=w179) -> ("设置文件内容结果"=→"设置文件内容结果":i32)  [unwired: 4 in, 2 out]
      }
      event "执行用例": Mouse Up {
        n117 = event-data() -> ()  [unwired: 1 in, 8 out]
        n118 = dll-call lib="D:/QuiKLab3.0/QuiKLabAPI.dll" fn="useTargetIp"(error in=w198, "指定IP"="192.168.1.222") -> (error out=w197:errorcluster, "设定使用下位机状态"=→"使用下位机返回值":i32)  [unwired: 3 in, 1 out]
        n119 = property on="用例分类" class="LstBox (严格)"() -> ("Item Names"=w192:string[], "Value"=w191:i32)  [unwired: 2 in, 2 out]
        n120 = property on="用例分类下用例" class="LstBox (严格)"() -> ("Item Names"=w189:string[], "Value"=w188:i32)  [unwired: 2 in, 2 out]
        n121 = Index Array(array=w192, index=w191) -> (element=w190:string)
        n122 = Index Array(array=w189, index=w188) -> (element=w187:string)
        n123 = dll-call lib="D:/QuiKLab3.0/QuiKLabAPI.dll" fn="useTestCase"(error in=w197, "用例集名"=w190, "用例名"=w187) -> (error out=w200:errorcluster, "useTestTask"=w185:i32)  [unwired: 4 in, 1 out]
        "useTestCase" <- w185
        n124 = Equal To 0?(x=w185) -> (x = 0?=w183:bool)
        n125 = dll-call lib="D:/QuiKLab3.0/QuiKLabAPI.dll" fn="startTestCase"(error in=w200, "测试记录名称"="1234" ("任务集名")) -> (error out=w181:errorcluster, "启动测试用例"=→"StartTest":i32)  [unwired: 3 in, 1 out]
        n126 = Select(t=T3."Enabled" ("Disable"), s=w183, f=T3."Disabled and Grayed Out" ("Disable")) -> (s? t:f=w180:T3)
        n127 = property on="停止测试用例" class="Bool"("DisabledEnum"=w180) -> ()  [unwired: 2 in, 2 out]
        n128 = property on="停止测试用例" class="Bool"("DisabledEnum"=w180) -> ()  [unwired: 2 in, 2 out]
        n129 = property on="设置文件内容" class="Bool"("DisabledEnum"=w180) -> ()  [unwired: 2 in, 2 out]
        n130 = property on="输出信号参数列表" class="Bool"("DisabledEnum"=w180) -> ()  [unwired: 2 in, 2 out]
        n131 = property on="输入信号参数列表" class="Bool"("DisabledEnum"=w180) -> ()  [unwired: 2 in, 2 out]
        n132 = dll-call lib="D:/QuiKLab3.0/QuiKLabAPI.dll" fn="unRegInputSignalParam"(error in=w181, "信号名"="signal" ("True"), "参数名"="P2") -> (error out=w195:errorcluster, "取消订阅"=→"取消订阅":i32)  [unwired: 4 in, 1 out]
      }
      event "发送信号": Mouse Up {
        n133 = event-data() -> ()  [unwired: 1 in, 8 out]
        n134 = dll-call lib="D:/QuiKLab3.0/QuiKLabAPI.dll" fn="sendOutputSignal"(error in=w205, "信号名"="signal" ("任务集名")) -> (error out=w204:errorcluster, "发送信号"=→"发送信号结果":i32)  [unwired: 3 in, 1 out]
      }
      event "暂停按钮": Mouse Up {
        n135 = event-data() -> ("CtlRef"=w210:refnum<vi>)  [unwired: 1 in, 1 out]
        n136 = property class="Bool (严格)"(reference=w210, error in=w211) -> (error out=w209:errorcluster, "Value"=w207:bool)  [unwired: 1 out]
        n137 = Boolean To (0,1)(Boolean=w207) -> (0, 1=w208:i16)
        n138 = dll-call lib="D:/QuiKLab3.0/QuiKLabAPI.dll" fn="setStatusIsPause"(error in=w209, "暂停和继续参数"=w208) -> (error out=w213:errorcluster, "暂停和继续结果"=→"暂停和继续结果":i32)  [unwired: 3 in, 1 out]
      }
      event "媒体停止按钮": Mouse Up {
        n139 = event-data() -> ()  [unwired: 1 in, 8 out]
        n140 = dll-call lib="D:/QuiKLab3.0/QuiKLabAPI.dll" fn="stopTestCase"(error in=w214) -> (error out=w215:errorcluster, "停止用例结果"=→"停止测试用例":i32)  [unwired: 2 in, 1 out]
      }
      event "退出程序": Mouse Up {
        n141 = event-data() -> ()  [unwired: 1 in, 8 out]
        n142 = dll-call lib="D:/QuiKLab3.0/QuiKLabAPI.dll" fn="stopTestTaskSet"(error in=w218) -> (error out=w219:errorcluster, "停止任务集结果"=→"停止任务集结果 2":i32)  [unwired: 2 in, 1 out]
        n143 = dll-call lib="D:/QuiKLab3.0/QuiKLabAPI.dll" fn="unLoadProject"(error in=w219) -> (error out=w224:errorcluster, "卸载工程结果"=→"卸载工程结果 2":i32)  [unwired: 2 in, 1 out]
        n144 = dll-call lib="D:/QuiKLab3.0/QuiKLabAPI.dll" fn="releaseQuiKLabPlatform"(error in=w224) -> (error out=w221:errorcluster, "释放平台结果"=→"释放平台结果":i32)  [unwired: 2 in, 1 out]
      }
      event "设置参数值": Mouse Up {
        n145 = event-data() -> ()  [unwired: 1 in, 8 out]
        n146 = property on="波形图表" class="WFChart (严格)"() -> ("Plot.Plot Name"=w225:string)  [unwired: 2 in, 2 out]
        n147 = dll-call lib="D:/QuiKLab3.0/QuiKLabAPI.dll" fn="setTestCaseRuntimeParamValue"(error in=w229, "参数名"=w225, "参数值"="设置实时参数值") -> (error out=w226:errorcluster, "设置参数值结果"=→"设置实时参数值返回值":i32)  [unwired: 4 in, 1 out]
      }
      event "设置输出信号参数值": Mouse Up {
        n148 = event-data() -> ()  [unwired: 1 in, 8 out]
        n149 = dll-call lib="D:/QuiKLab3.0/QuiKLabAPI.dll" fn="setOutputSignalParamValue"(error in=w236, "信号名"="signal", "参数名"="parameter_2", "参数值"="输出信号参数值") -> (error out=w234:errorcluster, "设置参数值结果"=→"设置输出参数值":i32, "参数值"=→"输出信号参数值":dbl)  [unwired: 4 in, 1 out]
      }
      event "设置初始值": Mouse Up {
        n150 = event-data() -> ()  [unwired: 1 in, 8 out]
        n151 = property on="获得初始值列表" class="MCListbox (严格)"() -> ("Value"=w237:i32, "ItemNames"=w241:string[][])  [unwired: 2 in, 2 out]
        n152 = property on="测试用例" class="LstBox (严格)"() -> ("Value"=w242:i32)  [unwired: 2 in, 2 out]
        n153 = Index Array(array=w241, index (row)=w237, index (col)=1 ("禁用的索引 (列)")) -> (element=w239:string)
        n154 = Decimal String To Number(string=w239) -> (number=w238:i32)  [unwired: 2 in, 1 out]
        n155 = dll-call lib="D:/QuiKLab3.0/QuiKLabAPI.dll" fn="setTestTaskTestCaseDoubleValue"(error in=w245, "用例索引"=w242, "初始值索引"=w237, "初始值"=w238) -> (error out=w243:errorcluster, "设置初始值值结果"=→"设置初始值结果":i32)  [unwired: 5 in, 1 out]
      }
      event "重置按钮": Mouse Up {
        n156 = event-data() -> ()  [unwired: 1 in, 8 out]
        n157 = dll-call lib="D:/QuiKLab3.0/QuiKLabAPI.dll" fn="resetInputSignal"(error in=w249, "信号名"="signal") -> (error out=w248:errorcluster, "重置参数值"=→"重置参数值":i32)  [unwired: 3 in, 1 out]
      }
      event "导出工程用例相关信息": Mouse Up {
        n158 = event-data() -> ()  [unwired: 1 in, 8 out]
        n159 = call "文件对话框"() -> ("selected path"=w254:path)  [unwired: 12 in, 3 out]
        n160 = Path To String(path=w254) -> (string=w252:string)
        n161 = dll-call lib="D:/QuiKLab3.0/QuiKLabAPI.dll" fn="exportTestCaseInfo"(error in=w250, "路径"=w252, "工程名"="1111-clone1" ("路径")) -> (error out=w251:errorcluster, "导出用例相关信息结果"=→"导出用例相关信息结果":i32)  [unwired: 4 in, 1 out]
      }
      event "加载工程": Mouse Up {
        n162 = control-ref of="卸载工程 2"() -> ()  [unwired: 1 out]
        n163 = event-data() -> ()  [unwired: 1 in, 8 out]
        n164 = property on="工程选择：" class="LstBox (严格)"() -> ("Item Names"=w260:string[], "Value"=w261:i32)  [unwired: 2 in, 2 out]
        n165 = Index Array(array=w260, index=w261) -> (element=w259:string)
        n166 = dll-call lib="D:/QuiKLab3.0/QuiKLabAPI.dll" fn="loadProject"(error in=w262, "工程名"=w259) -> (error out=w258:errorcluster, "加载工程结果"=w257:i32)  [unwired: 3 in, 1 out]
        "加载工程结果" <- w257
        n167 = Equal To 0?(x=w257) -> (x = 0?=w256:bool)
        n168 = case shown="真" w256 {
          frame False {
          }
          frame True {
            w263 = T3."Enabled" ("Disable")
            n169 = property on="加载工程" class="Bool"("DisabledEnum"=T3."Disabled and Grayed Out" ("Disable")) -> ()  [unwired: 2 in, 2 out]
            n170 = property on="更新路径" class="Bool"("DisabledEnum"=w263) -> ()  [unwired: 2 in, 2 out]
            n171 = property on="导出工程用例相关信息" class="Bool"("DisabledEnum"=w263) -> ()  [unwired: 2 in, 2 out]
            n172 = property on="执行用例" class="Bool"("DisabledEnum"=w263) -> ()  [unwired: 2 in, 2 out]
            n173 = property on="卸载工程" class="Bool"("DisabledEnum"=w263) -> ()  [unwired: 2 in, 2 out]
            n174 = property on="播放按钮" class="Bool"("DisabledEnum"=w263) -> ()  [unwired: 2 in, 2 out]
            n175 = property on="输入信号参数列表" class="Bool"("DisabledEnum"=w263) -> ()  [unwired: 2 in, 2 out]
            n176 = property on="设置文件内容" class="Bool"("DisabledEnum"=w263) -> ()  [unwired: 2 in, 2 out]
            n177 = property on="输出信号参数列表" class="Bool"("DisabledEnum"=w263) -> ()  [unwired: 2 in, 2 out]
          }
        }
      }
      event "下位机信息": Mouse Up {
        n178 = event-data() -> ()  [unwired: 1 in, 8 out]
        n179 = dll-call lib="D:/QuiKLab3.0/QuiKLabAPI.dll" fn="getTargetCount"(error in=w275) -> (error out=w274:errorcluster, "返回类型"=w276:i32)  [unwired: 2 in, 1 out]
        "下位机个数" <- w276
        n180 = for {
          N: w276 -> [_]
          shift-right: [w301] -> w265
          shift-left: w274 -> [w293]
          tunnel: [w294] -> w273 mode=indexing
          i -> [w300]
          n181 = local read "字符串 3"() -> (w299:string)
          n182 = String Length(string=w299) -> (length=w298:i32)
          n183 = dll-call lib="D:/QuiKLab3.0/QuiKLabAPI.dll" fn="getTargetIP"(error in=w293, "索引"=w300, "IP值"=w299, "IP长度"=w298) -> (error out=w301:errorcluster, "IP值"=w292:string)  [unwired: 5 in, 1 out]
          n184 = dll-call lib="D:/QuiKLab3.0/QuiKLabAPI.dll" fn="getTargetState"("下位机IP"=w292) -> ("返回下位机状态"=w296:i32)  [unwired: 4 in, 2 out]
          n185 = Number To Decimal String(number=w296, width (-)=i16 0 ("宽度(-)")) -> (decimal integer string=w297:string)
          n186 = Build Array ("创建数组")(w292, w297) -> (w294:string[])
        }
        n187 = property on="下位机列表" class="MCListbox (严格)"("ItemNames"=w273) -> ()  [unwired: 2 in, 2 out]
        n188 = dll-call lib="D:/QuiKLab3.0/QuiKLabAPI.dll" fn="getIpState"(error in=w265, "设备IP"="输入设备IP") -> (error out=w279:errorcluster, "返回IP是否在线"=→"IP是否在线":i32)  [unwired: 3 in, 1 out]
        n189 = dll-call lib="D:/QuiKLab3.0/QuiKLabAPI.dll" fn="updateInterfInfos"(error in=w279) -> (error out=w277:errorcluster, "返回是否成功"=→"更新信息是否成功":i32)  [unwired: 2 in, 1 out]
        n190 = dll-call lib="D:/QuiKLab3.0/QuiKLabAPI.dll" fn="getInterfNumFromIp"(error in=w277, "设备IP"="板卡设备IP") -> (error out=w271:errorcluster, "板卡类型个数"=w269:i32, "设备IP"=w267:string)  [unwired: 2 in, 1 out]
        "板卡类型个数" <- w269
        n191 = for {
          N: w269 -> [_]
          shift-right: [w287] -> w270
          shift-left: w271 -> [w286]
          tunnel: [w282] -> w268 mode=indexing
          tunnel: w267 -> [w281]
          i -> [w285]
          w289 = "0000000000000000000000" ("板卡信息")
          w288 = "000000000000000000000000000000000000000000000000" ("板卡名称")
          n192 = String Length(string=w289) -> (length=w291:i32)
          n193 = String Length(string=w288) -> (length=w290:i32)
          n194 = dll-call lib="D:/QuiKLab3.0/QuiKLabAPI.dll" fn="getInterfInfo"(error in=w286, "设备IP"=w281, "板卡索引"=w285, "板卡名称"=w288, "板卡名称长度"=w290, "板卡信息"=w289, "板卡信息长度"=w291) -> (error out=w287:errorcluster, "板卡名称"=w284:string, "板卡信息"=w283:string)  [unwired: 7 in, 1 out]
          n195 = Build Array ("创建数组")(w284, w283) -> (w282:string[])
        }
        n196 = property on="板卡信息列表" class="MCListbox (严格)"("ItemNames"=w268) -> ()  [unwired: 2 in, 2 out]
      }
      event "卸载工程": Mouse Up {
        n197 = event-data() -> ()  [unwired: 1 in, 8 out]
        n198 = dll-call lib="D:/QuiKLab3.0/QuiKLabAPI.dll" fn="unLoadProject"(error in=w315) -> (error out=w314:errorcluster, "卸载工程结果"=w313:i32)  [unwired: 2 in, 1 out]
        "卸载工程结果" <- w313
        n199 = Equal To 0?(x=w313) -> (x = 0?=w312:bool)
        n200 = call "初始化 (子VI).vi"("Boolean输入"=w311, "卸载工程"=w309, "设置文件内容"=w310, "布尔"=w312, "更新路径"=w308, "停止测试用例"=w307, "导出工程用例相关信息"=w306, "播放按钮"=w305, "暂停按钮"=w304, "媒体停止按钮"=w303, "执行用例"=w302) -> ()  [unwired: 5 in]
      }
      event "更新路径": Mouse Up {
        n201 = event-data() -> ()  [unwired: 1 in, 8 out]
        n202 = dll-call lib="D:/QuiKLab3.0/QuiKLabAPI.dll" fn="updateTestTaskSetTablePath"(error in=w317, "任务集表路径"="E:\\testtaskset.xml") -> (error out=w316:errorcluster, "更新路径结果"=→"更新路径结果":i32)  [unwired: 3 in, 1 out]
      }
      event "获取任务集列表": Mouse Up {
        n203 = event-data() -> ()  [unwired: 1 in, 8 out]
        n204 = invoke on="任务集" class="Tree (严格)" method="Edit Tree Items.Delete"(error in=w330) -> (error out=w329:errorcluster)  [unwired: 4 in, 4 out]
        n205 = dll-call lib="D:/QuiKLab3.0/QuiKLabAPI.dll" fn="getTestTaskClassCount"(error in=w329) -> (error out=w328:errorcluster, "任务集数量"=w331:i32)  [unwired: 2 in, 1 out]
        n206 = for {
          N: w331 -> [_]
          shift-right: [w338] -> w327
          shift-left: w328 -> [_]
          tunnel: [w337] -> w326 mode=indexing
          i -> [w346]
          w345 = "00000000000000" ("任务集名称")
          n207 = String Length(string=w345) -> (length=w344:i32)
          n208 = dll-call lib="D:/QuiKLab3.0/QuiKLabAPI.dll" fn="getTestTaskClassName"("任务集索引"=w346, "任务集名称"=w345, "长度"=w344) -> (error out=w343:errorcluster, "任务集名称"=w337:string)  [unwired: 6 in, 1 out]
          n209 = invoke on="任务集" class="Tree (严格)" method="Edit Tree Items.Add Item to End"(error in=w343, "Left Cell"=w337) -> (error out=w342:errorcluster)  [unwired: 6 in, 7 out]
          n210 = dll-call lib="D:/QuiKLab3.0/QuiKLabAPI.dll" fn="getTestTaskCount"(error in=w342, "任务集名称"=w337) -> (error out=w339:errorcluster, "获取任务数量"=w341:i32, "任务集名称"=w340:string)  [unwired: 2 in, 1 out]
          n211 = for {
            N: w341 -> [_]
            tunnel: w340 -> [w351]
            shift-right: [w348] -> w338
            shift-left: w339 -> [w350]
            i -> [w347]
            w354 = "000000000000000000000000000" ("任务名称")
            n212 = String Length(string=w354) -> (length=w353:i32)
            n213 = dll-call lib="D:/QuiKLab3.0/QuiKLabAPI.dll" fn="getTestTaskName"(error in=w350, "任务集名称"=w351, "任务索引"=w347, "任务名称"=w354, "长度"=w353) -> (error out=w349:errorcluster, "任务名称"=w352:string)  [unwired: 6 in, 1 out]
            n214 = invoke on="任务集" class="Tree (严格)" method="Edit Tree Items.Add Item"(error in=w349, "Parent Tag"=w351, "Child Position"=w347, "Left Cell"=w352) -> (error out=w348:errorcluster)  [unwired: 5 in, 8 out]
          }
        }
        n215 = property on="测试任务" class="LstBox (严格)"() -> ("Item Names"=w325:string[], "Value"=w324:i32)  [unwired: 2 in, 2 out]
        n216 = property on="测试任务" class="LstBox (严格)"("Item Names"=w326) -> ()  [unwired: 2 in, 2 out]
        n217 = Index Array(array=w325, index=w324) -> (element=w323:string)
        n218 = dll-call lib="D:/QuiKLab3.0/QuiKLabAPI.dll" fn="getTestTaskCount"("任务集名称"=w323) -> ("获取任务数量"=w322:i32, "任务集名称"=w321:string)  [unwired: 3 in, 2 out]
        n219 = for {
          N: w322 -> [_]
          tunnel: w321 -> [w335]
          tunnel: [w334] -> w320 mode=indexing
          i -> [w336]
          w333 = "0000000000000000000000000000" ("任务名称")
          n220 = String Length(string=w333) -> (length=w332:i32)
          n221 = dll-call lib="D:/QuiKLab3.0/QuiKLabAPI.dll" fn="getTestTaskName"("任务集名称"=w335, "任务索引"=w336, "任务名称"=w333, "长度"=w332) -> ("任务名称"=w334:string)  [unwired: 7 in, 2 out]
        }
        n222 = property on="任务分类下任务" class="LstBox (严格)"("Item Names"=w320) -> ()  [unwired: 2 in, 2 out]
      }
      event "输入信号参数列表": Mouse Up {
        n223 = event-data() -> ()  [unwired: 1 in, 8 out]
        n224 = invoke on="输入信号列表" class="Tree (严格)" method="Edit Tree Items.Delete"(error in=w358) -> (error out=w357:errorcluster)  [unwired: 4 in, 4 out]
        n225 = dll-call lib="D:/QuiKLab3.0/QuiKLabAPI.dll" fn="getInputSignalCount"(error in=w357) -> (error out=w356:errorcluster, "输入信号数量"=w359:i32)  [unwired: 2 in, 1 out]
        n226 = for {
          N: w359 -> [_]
          shift-right: [w366] -> w355
          shift-left: w356 -> [w365]
          i -> [w375]
          w374 = "00000000000000" ("任务集名称")
          n227 = String Length(string=w374) -> (length=w373:i32)
          n228 = dll-call lib="D:/QuiKLab3.0/QuiKLabAPI.dll" fn="getInputSignalName"(error in=w365, "信号索引"=w375, "输入信号名称"=w374, "长度"=w373) -> (error out=w371:errorcluster, "输入信号名称"=w372:string)  [unwired: 5 in, 1 out]
          n229 = invoke on="输入信号列表" class="Tree (严格)" method="Edit Tree Items.Add Item to End"(error in=w371, "Left Cell"=w372) -> (error out=w370:errorcluster)  [unwired: 6 in, 7 out]
          n230 = dll-call lib="D:/QuiKLab3.0/QuiKLabAPI.dll" fn="getSignalParamCount"(error in=w370, "信号名"=w372) -> (error out=w367:errorcluster, "获取信号参数数量"=w369:i32, "信号名"=w368:string)  [unwired: 2 in, 1 out]
          n231 = for {
            N: w369 -> [_]
            tunnel: w368 -> [w380]
            shift-right: [w377] -> w366
            shift-left: w367 -> [w379]
            i -> [w376]
            w383 = "0000000000000" ("任务名称")
            n232 = String Length(string=w383) -> (length=w382:i32)
            n233 = dll-call lib="D:/QuiKLab3.0/QuiKLabAPI.dll" fn="getSignalParamName"(error in=w379, "信号名称"=w380, "信号索引"=w376, "参数名称"=w383, "长度"=w382) -> (error out=w378:errorcluster, "参数名称"=w381:string)  [unwired: 6 in, 1 out]
            n234 = invoke on="输入信号列表" class="Tree (严格)" method="Edit Tree Items.Add Item"(error in=w378, "Parent Tag"=w380, "Child Position"=w376, "Left Cell"=w381) -> (error out=w377:errorcluster)  [unwired: 5 in, 8 out]
          }
        }
        n235 = disable-structure shown="禁用" {
          frame Disabled {
            n236 = invoke on="输入信号列表" class="Tree (严格)" method="Double Click"() -> ("Double Click"=w361:string)  [unwired: 3 in, 2 out]
            n237 = Empty String/Path?(string/path=w361) -> (empty?=w360:bool)
            n238 = case shown="假" w360 {
              frame False {
                n239 = invoke on="输入信号列表" class="Tree (严格)" method="Double Click"() -> ("Double Click"=w362:string)  [unwired: 3 in, 2 out]
                "双击" <- w362
                n240 = invoke on="输入信号列表" class="Tree (严格)" method="Navigate Tree.Get Parent"("tag"=w362) -> ("Navigate Tree:Get Parent"=w364:string)  [unwired: 3 in, 3 out]
                "信号" <- w364
                n241 = dll-call lib="D:/QuiKLab3.0/QuiKLabAPI.dll" fn="getInputSignalParamValue"("信号名"=w364, "参数名"=w362) -> ("获取订阅的信号参数值"=→"获取订阅的信号参数值":dbl)  [unwired: 5 in, 2 out]
              }
              frame True {
              }
            }
          }
          frame Enabled {
          }
        }
      }
      event "输出信号参数列表": Mouse Up {
        n242 = event-data() -> ()  [unwired: 1 in, 8 out]
        n243 = invoke on="输出信号列表" class="Tree (严格)" method="Edit Tree Items.Delete"(error in=w387) -> (error out=w386:errorcluster)  [unwired: 4 in, 4 out]
        n244 = dll-call lib="D:/QuiKLab3.0/QuiKLabAPI.dll" fn="getOutputSignalCount"(error in=w386) -> (error out=w385:errorcluster, "输入信号数量"=w388:i32)  [unwired: 2 in, 1 out]
        n245 = for {
          N: w388 -> [_]
          shift-right: [w390] -> w384
          shift-left: w385 -> [w389]
          i -> [w399]
          w398 = "00000000000000" ("任务集名称")
          n246 = String Length(string=w398) -> (length=w397:i32)
          n247 = dll-call lib="D:/QuiKLab3.0/QuiKLabAPI.dll" fn="getOutputSignalName"(error in=w389, "信号索引"=w399, "输入信号名称"=w398, "长度"=w397) -> (error out=w395:errorcluster, "输入信号名称"=w396:string)  [unwired: 5 in, 1 out]
          n248 = invoke on="输出信号列表" class="Tree (严格)" method="Edit Tree Items.Add Item to End"(error in=w395, "Left Cell"=w396) -> (error out=w394:errorcluster)  [unwired: 6 in, 7 out]
          n249 = dll-call lib="D:/QuiKLab3.0/QuiKLabAPI.dll" fn="getSignalParamCount"(error in=w394, "信号名"=w396) -> (error out=w391:errorcluster, "获取信号参数数量"=w393:i32, "信号名"=w392:string)  [unwired: 2 in, 1 out]
          n250 = for {
            N: w393 -> [_]
            tunnel: w392 -> [w404]
            shift-right: [w401] -> w390
            shift-left: w391 -> [w403]
            i -> [w400]
            w407 = "0000000000000" ("任务名称")
            n251 = String Length(string=w407) -> (length=w406:i32)
            n252 = dll-call lib="D:/QuiKLab3.0/QuiKLabAPI.dll" fn="getSignalParamName"(error in=w403, "信号名称"=w404, "信号索引"=w400, "参数名称"=w407, "长度"=w406) -> (error out=w402:errorcluster, "参数名称"=w405:string)  [unwired: 6 in, 1 out]
            n253 = invoke on="输出信号列表" class="Tree (严格)" method="Edit Tree Items.Add Item"(error in=w402, "Parent Tag"=w404, "Child Position"=w400, "Left Cell"=w405) -> (error out=w401:errorcluster)  [unwired: 5 in, 8 out]
          }
        }
      }
      event "获取用例集列表": Mouse Up {
        n254 = event-data() -> ()  [unwired: 1 in, 8 out]
        n255 = invoke on="用例集" class="Tree (严格)" method="Edit Tree Items.Delete"(error in=w419) -> (error out=w418:errorcluster)  [unwired: 4 in, 4 out]
        n256 = dll-call lib="D:/QuiKLab3.0/QuiKLabAPI.dll" fn="getTestCaseClassCount"(error in=w418) -> (error out=w416:errorcluster, "获取用例集数量"=w417:i32)  [unwired: 2 in, 1 out]
        n257 = for {
          N: w417 -> [_]
          shift-right: [w426] -> w415
          shift-left: w416 -> [w431]
          tunnel: [w425] -> w414 mode=indexing
          i -> [w435]
          w433 = "0000000000000000000000" ("用例集名称")
          n258 = String Length(string=w433) -> (length=w434:i32)
          n259 = dll-call lib="D:/QuiKLab3.0/QuiKLabAPI.dll" fn="getTestCaseClassName"(error in=w431, "用例集索引"=w435, "用例集名称"=w433, "长度"=w434) -> (error out=w430:errorcluster, "用例集名称"=w425:string)  [unwired: 5 in, 1 out]
          n260 = invoke on="用例集" class="Tree (严格)" method="Edit Tree Items.Add Item to End"(error in=w430, "Left Cell"=w425) -> (error out=w429:errorcluster)  [unwired: 6 in, 7 out]
          n261 = dll-call lib="D:/QuiKLab3.0/QuiKLabAPI.dll" fn="getTestCaseCount"(error in=w429, "用例集名称"=w425) -> (error out=w428:errorcluster, "获取用例数量"=w432:i32, "用例集名称"=w427:string)  [unwired: 2 in, 1 out]
          n262 = for {
            N: w432 -> [_]
            shift-right: [w441] -> w426
            shift-left: w428 -> [w438]
            tunnel: w427 -> [w437]
            i -> [w436]
            w442 = "0000000000000000000000000" ("用例名称")
            n263 = String Length(string=w442) -> (length=w443:i32)
            n264 = dll-call lib="D:/QuiKLab3.0/QuiKLabAPI.dll" fn="getTestCaseName"(error in=w438, "用例集名称"=w437, "用例索引"=w436, "用例名称"=w442, "长度"=w443) -> (error out=w439:errorcluster, "用例名称"=w440:string)  [unwired: 6 in, 1 out]
            n265 = invoke on="用例集" class="Tree (严格)" method="Edit Tree Items.Add Item"(error in=w439, "Parent Tag"=w437, "Child Position"=w436, "Left Cell"=w440) -> (error out=w441:errorcluster)  [unwired: 5 in, 8 out]
          }
        }
        n266 = property on="用例分类" class="LstBox (严格)"("Item Names"=w414) -> ()  [unwired: 2 in, 2 out]
        n267 = property on="用例分类" class="LstBox (严格)"() -> ("Item Names"=w413:string[], "Value"=w412:i32)  [unwired: 2 in, 2 out]
        n268 = Index Array(array=w413, index=w412) -> (element=w411:string)
        n269 = dll-call lib="D:/QuiKLab3.0/QuiKLabAPI.dll" fn="getTestCaseCount"("用例集名称"=w411) -> ("获取用例数量"=w410:i32, "用例集名称"=w409:string)  [unwired: 3 in, 2 out]
        n270 = for {
          N: w410 -> [_]
          tunnel: w409 -> [w423]
          tunnel: [w422] -> w408 mode=indexing
          i -> [w424]
          w421 = "00000000000000000000000000000000" ("用例名称")
          n271 = String Length(string=w421) -> (length=w420:i32)
          n272 = dll-call lib="D:/QuiKLab3.0/QuiKLabAPI.dll" fn="getTestCaseName"("用例集名称"=w423, "用例索引"=w424, "用例名称"=w421, "长度"=w420) -> ("用例名称"=w422:string)  [unwired: 7 in, 2 out]
        }
        n273 = property on="用例分类下用例" class="LstBox (严格)"("Item Names"=w408) -> ()  [unwired: 2 in, 2 out]
      }
      event "获得初始值": Mouse Up {
        n274 = event-data() -> ()  [unwired: 1 in, 8 out]
        n275 = dll-call lib="D:/QuiKLab3.0/QuiKLabAPI.dll" fn="getTestTaskTestCaseCount"(error in=w450) -> (error out=w447:errorcluster, "测试任务下用例数量"=w449:i32)  [unwired: 2 in, 1 out]
        n276 = for {
          N: w449 -> [_]
          tunnel: [w457] -> w448 mode=indexing
          shift-right: [w455] -> w446
          shift-left: w447 -> [w456]
          i -> [w460]
          n277 = dll-call lib="D:/QuiKLab3.0/QuiKLabAPI.dll" fn="getTestTaskTestCaseName"(error in=w456, "用例索引"=w460, "测试用例名"="000000000000000000000000000", "长度"=100) -> (error out=w455:errorcluster, "测试用例名"=w457:string)  [unwired: 5 in, 1 out]
        }
        n278 = property on="测试用例" class="LstBox (严格)"("Item Names"=w448) -> ()  [unwired: 2 in, 2 out]
        n279 = property on="测试用例" class="LstBox (严格)"() -> ("Value"=w445:i32)  [unwired: 2 in, 2 out]
        n280 = dll-call lib="D:/QuiKLab3.0/QuiKLabAPI.dll" fn="getTestTaskTestCaseDoubleCount"(error in=w446, "用例索引"=w445) -> (error out=w453:errorcluster, "初始值数量"=w454:i32, "用例索引"=w451:i32)  [unwired: 2 in, 1 out]
        n281 = for {
          N: w454 -> [_]
          shift-right: [w468] -> w444
          shift-left: w453 -> [w467]
          tunnel: [w462] -> w452 mode=indexing
          tunnel: w451 -> [w461]
          i -> [w469]
          w470 = "000000000000000000" ("参数名称")
          n282 = String Length(string=w470) -> (length=w471:i32)
          n283 = dll-call lib="D:/QuiKLab3.0/QuiKLabAPI.dll" fn="getTestTaskTestCaseDoubleNameValue"(error in=w467, "用例索引"=w461, "初始值索引"=w469, "初始名"=w470, "初始名长度"=w471) -> (error out=w468:errorcluster, "初始名"=w463:string, "初始值"=w464:dbl)  [unwired: 7 in, 1 out]
          n284 = Number To Decimal String(number=w464, width (-)=i16 0) -> (decimal integer string=w465:string)
          n285 = Build Array ("创建数组")(w463, w465) -> (w462:string[])
        }
        n286 = property on="获得初始值列表" class="MCListbox (严格)"("ItemNames"=w452) -> ()  [unwired: 2 in, 2 out]
      }
    }
  }
